vi "AMSClient.vi"() -> ()   [LabVIEW 2013]
uses:
  Controls/DB - Logon Info.ctl
  Controls/DB - Logon Extra Info.ctl
  Controls/Combo Box.ctl
  Controls/Enum - CMS State.ctl
  <vilib>/Utility/miscctls.llb/LVPointTypeDef.ctl
  <vilib>/Utility/miscctls.llb/LVRowAndColumnUnsignedTypeDef.ctl
  <vilib>/Utility/miscctls.llb/LVRowAndColumnTypeDef.ctl
  Controls/DB - [AMS].[Execute].[Message] ColNames.ctl
  <vilib>/Utility/miscctls.llb/LVDateTimeRec.ctl
  Controls/DB - [AMS].[Execute].[Message] Enum.ctl
  <vilib>/Utility/NIReport.llb/NI_report.lvclass
  Controls/DB - OpenClose.ctl
  Controls/DB - [AMS].[Execute].[EventLog] Enum.ctl
  Controls/DB - AMS Execute EventLog.ctl
  Controls/Global AMS.vi
  <vilib>/Utility/NIReport.llb/Append Text Table to Report (wrap).vi
  Controls/Global CMS.vi
  <vilib>/Utility/config.llb/Write Key (String).vi
  Controls/Message Code - Enum.ctl
  Controls/Enum - SRTRS State.ctl
  <vilib>/Utility/config.llb/NI_LVConfig.lvlib
panel:
  in  "Tab Footer":enum32{"Page 1"}(tab) caption="Tab Header"
  out "Current Time":string
  in  "Tab Header":enum32{"Page 1"}(tab)
  out "LogoName":picture
  in  "Close":bool
  out "Plant and Furnace Name":string="OneSubsea, Johor / BH0277."
  out "ApplicationName":string caption="[LogoName]"
  in  "Tab Body":T1(tab)=enum."Logon"
  out "Last Alive On":string
  out "Overall Status":bool caption="Engine Status"
  in  "Search":bool caption="Setup Save"
  in  "Max Record to Display":i32 caption="Max. Records To Display"
  in  "Ref Message No":string caption="Ref. Message No."
  in  "Message No":string caption="Message No."
  in  "Plant":T2
  in  "Email":T2
  in  "SMS":T2
  in  "Application ComboBox":T2 caption="Application"
  in  "To Date":timestamp caption="To" format="%<%Y-%m-%d>T"
  in  "From Date":timestamp caption="From" format="%<%Y-%m-%d>T"
  in  "Criteria [CaptionOnly]":string caption="Criteria"
  in  "Resend":bool caption="Setup Save"
  in  "Reprocess [CaptionOnly]":string caption="Reprocess"
  in  "Excel":bool caption="Setup Save"
  in  "Export To [CaptionOnly]":string caption="Export To"
  in  "List [CaptionOnly]":string caption="List"
  in  "Multicolumn Listbox":i32[](listbox)
  in  "MyTab":T3(tab)
  out "Toggle Search":bool=TRUE
  out "Property":errorcluster
  in  "CellBG Unused Cells":u32(colorbox)=16777238
  in  "CellBG ColHdrs":u32(colorbox)=11776947
  in  "Ascending":bool
  out "<CONDITIONS>":string="[MessageNo] >0"
  out "EnginePollIntInSec":i32
  in  "Time Target (s)":dbl=1.0
  out "Engine Alive":timestamp format="%<%I:%M:%S%3u %p\n%x>T"
  out "Engine Start":timestamp format="%<%I:%M:%S%3u %p\n%x>T"
  out "Engine Stop":timestamp format="%<%I:%M:%S%3u %p\n%x>T"
  out "Report":errorcluster
  out "Toggle Refresh MCListBox Colors":bool=TRUE
  out "Metrics:Code Size":u32=1762288 format="%#.3p"
  out "SubPanel Error":errorcluster
  out "Logon OK":bool
  in  "[TabUserAccess]":bool[](array[boolean])=[FALSE, FALSE, FALSE, FALSE, FALSE, FALSE, FALSE, FALSE, FALSE, FALSE, FALSE, FALSE, FALSE, FALSE, FALSE, FALSE, FALSE, FALSE, FALSE, FALSE]
  in  "Logon Extra":T4
  in  "Logon":T5
  out "Current VI's path":path
  out "Front Panel Window:State":T6(ring)
  out "Execution:State":T7(ring)
  out "Admin User UI":refnum<vi>
  out "Logon UI":refnum<vi>
  out "Config UI":refnum<vi>
  in  "Application":string="AMS"
  out "Max Rec to Display (Startup)":i32
  out "ini File":errorcluster
  out "LogonName Error":errorcluster
  out "Station":string
  out "Plant":string
  out "LabVIEW Directory Path":path
  out "Application:Name":string="LabVIEW.exe"
  out "[TimeZone] (Plant)":string
  out "[CmsServerTz] (CMS)":string
  out "TimeZone Diff (NA)":i32
  out "Plant and Furnace Name (B4 Logon)":string="OneSubsea, Johor / BH0277." caption="Plant and Furnace Name"
  out "Application Directory":path=path "C:/Users/CK/workspace/LabVIEW/Stress Relief Temperature Recording"
  out "Error Out":errorcluster
  out "Show Debug TAB":bool=TRUE caption="Show Debug Tab"
  out "Quit Flag":bool
  out "Close Flag":bool=TRUE
  out "Summary":errorcluster
  out "MHandler":errorcluster
  in  "DB - Logon":bool=TRUE
  out "File Version":string
  in  "Debug Close":bool caption="Close"
  # "User Details"
  # "System Status"
  # "Logon"
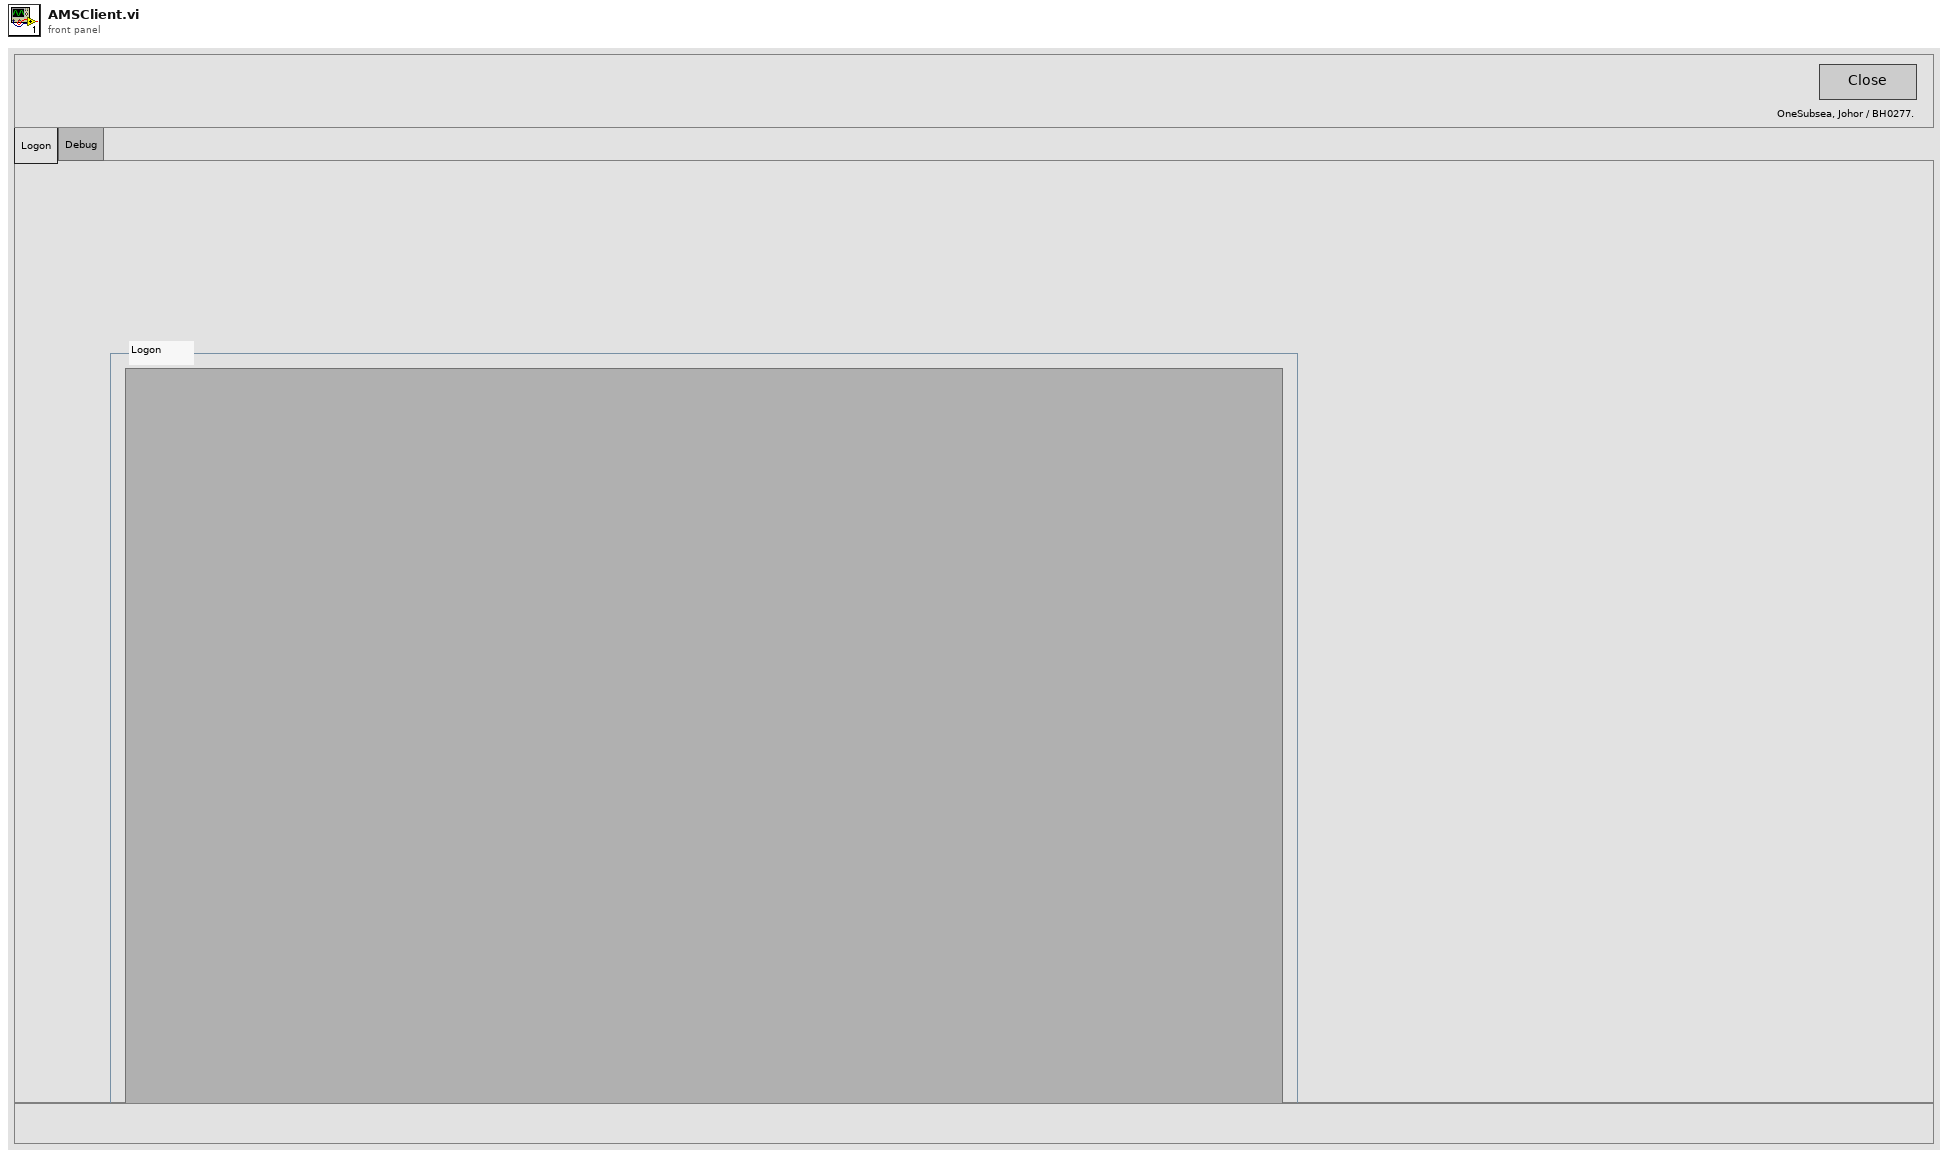
[diagram p1: front panel]
types:
  T1 = enum32{"Monitor", "Admin", "Config", "Logon", "Debug"}
  T2 = typedef "Combo Box.ctl" = string
  T3 = enum32{"Monitor", "SubPanel", "Settings", "Others", "DB"}
  T4 = typedef "DB - Logon Extra Info.ctl" = cluster{"Plant Name":string, "UserName":string, "Hostname [ClientName]":string, "IsUnicode":bool}
  T5 = typedef "DB - Logon Info.ctl" = cluster{"PlantID":string, "SystemID":string, "UserID":string, "DomainID":string, "LanguageID":string, "StationID":string}
  T6 = enum32{"Invalid", "Standard", "Closed", "Hidden", "Minimized", "Maximized"}
  T7 = enum32{"Bad", "Idle", "Run top level", "Running"}
  T8 = typedef "Enum - CMS State.ctl" = enum16{"READY TO START", "RUNNING Process", "QUIT"}
  T9 = enum16{"Always On", "Always Off", "Off While Running"}
  T10 = typedef "LVRowAndColumnUnsignedTypeDef.ctl" = cluster{"Row":u32, "Column":u32}
  T11 = typedef "LVPointTypeDef.ctl" = cluster{"Horizontal":i16, "Vertical":i16}
  T12 = typedef "DB - [AMS].[Execute].[Message] ColNames.ctl" = enum16{"[MessageNo]", "[LanguageId]", "[SoftwareSolutionId]", "[SoftwareSolutionName]", "[PlantId]", "[SystemId]", "[StationId]", "[MessageLogNo]", "[ReceivedOn]", "[MessageCode]", "[ShortDescription]", "[Message]", "[SmsMessage]", "[SuppMessage1]", "[SuppMessage2]", "[SuppMessage3]", "[TransactionNo]", "[TransactionRunNo]", "[MessageInitiator]", "[Remarks]", "[MsgCreatedOn]", "[IsToSendSms]", "[IsToSendEmail]", "[IsToSendCommMedium1]", "[IsToSendCommMedium2]", "[SmsContent]", "[EmailContent]", "[CommMed1Content]", "[CommMed2Content]", "[MobileNos]", "[EmailAddresses]", "[CommMedium1Ids]", "[CommMedium2Ids]", "[LastAttemptedCommMed]", "[LastAttemptedNo]", "[LastAttemptedOn]", "[IsSmsSent]", "[IsEmailSent]", "[IsCommMedium1Sent]", "[IsCommMedium2Sent]", "[OverallSentStatus]", "[StatusUpdatedOn]", "[IsArchived]"}
  T13 = typedef "LVRowAndColumnTypeDef.ctl" = cluster{"Row":i32, "Column":i32}
  T14 = cluster{"LogoFile":string, "Software Solution Name":string}
  T15 = typedef "Connection Information Cluster.ctl" = cluster{"Connection ":string, "Username":string, "Password":string}
  T16 = cluster{"Show LabVIEW Error":bool, "Show Debug Tab":bool, "Show Scrollbars":bool}
  T17 = typedef "imagedata.ctl" = cluster{"image type":i32, "image depth":i32, "image":u8[], "mask":u8[], "colors":u32[], "Rectangle":cluster{"left":i16, "top":i16, "right":i16, "bottom":i16}}
  T18 = typedef "Enum - SRTRS State.ctl" = enum16{"READY TO START", "START Recipe", "START Recovery", "BEGIN Process", "RUNNING Process", "END Process", "Spare Enum", "END Recipe", "ERROR Handling", "QUIT"}
  T19 = typedef "Message Code - Enum.ctl" = enum16{"<APP><I 100>", "<APP><E 101>", "<APP><I 110>", "<APP><W 111>", "<APP><I 112>", "<APP><W 113>", "<APP><I 114>", "<APP><I 115>", "<APP><I 116>", "<APP><W 117>", "<APP><I 120>", "<APP><W 121>", "<APP><E 122>", "<APP><W 130>", "<APP><W 131>", "<APP><W 132>", "<APP><W 133>", "<APP><W 134>", "<DB><I 150>", "<DB><I 151>", "<DB><W 152>", "<APP><I 200>", "<APP><I 201>", "<APP><W 202>", "<APP><E 203>", "<DB><I 300>", "<DB><I 301>", "<DB><W 302>", "<DB><I 305>", "<DB><I 306>", "<DB><W 307>", "<DB><W 310>", "<cRIO><I 400>", "<cRIO><W 401>", "<cRIO><I 402>", "<cRIO><W 403>", "<ET><I 500>", "<ET><W 501>", "<ET><I 600>", "<ET><W 601>", "<ET><E 602>", "<ET><I 610>", "<ET><W 611>", "<ET><E 612>"}
  T20 = typedef "DB - [AMS].[Execute].[Message] Enum.ctl" = enum16{"SELECT", "SELECT (Multi-Conditions)", "UPDATE", "RE-INSERT"}
  T21 = enum16{"maximized", "minimized", "normal", "no change"}
  T22 = enum16{"Standard Report", "HTML", "Word", "Excel"}
  T23 = typedef "LVDateTimeRec.ctl" = cluster{"fractional second":dbl, "second":i32, "minute":i32, "hour":i32, "day of month":i32, "month":i32, "year":i32, "day of week":i32, "day of year":i32, "DST":i32}
  T24 = typedef "DB - AMS Execute EventLog.ctl" = cluster{"EventType":string, "Source":string, "UserId":string, "Computer":string, "CreatedOn":string, "Remarks1":string}
  T25 = typedef "DB - OpenClose.ctl" = cluster{"Open":bool, "Close":bool}
  T26 = typedef "NI_LVConfig.lvlib/Config Data RefNum.ctl" = refnum<k1>
  T27 = typedef "DB - [AMS].[Execute].[EventLog] Enum.ctl" = enum16{"SELECT 'CreatedOn'", "SELECT 'LastMessageNo'", "INSERT"}
  T28 = typedef "NI_Database_API.lvlib/Conn ObjectReference.ctl" = refnum<k1>
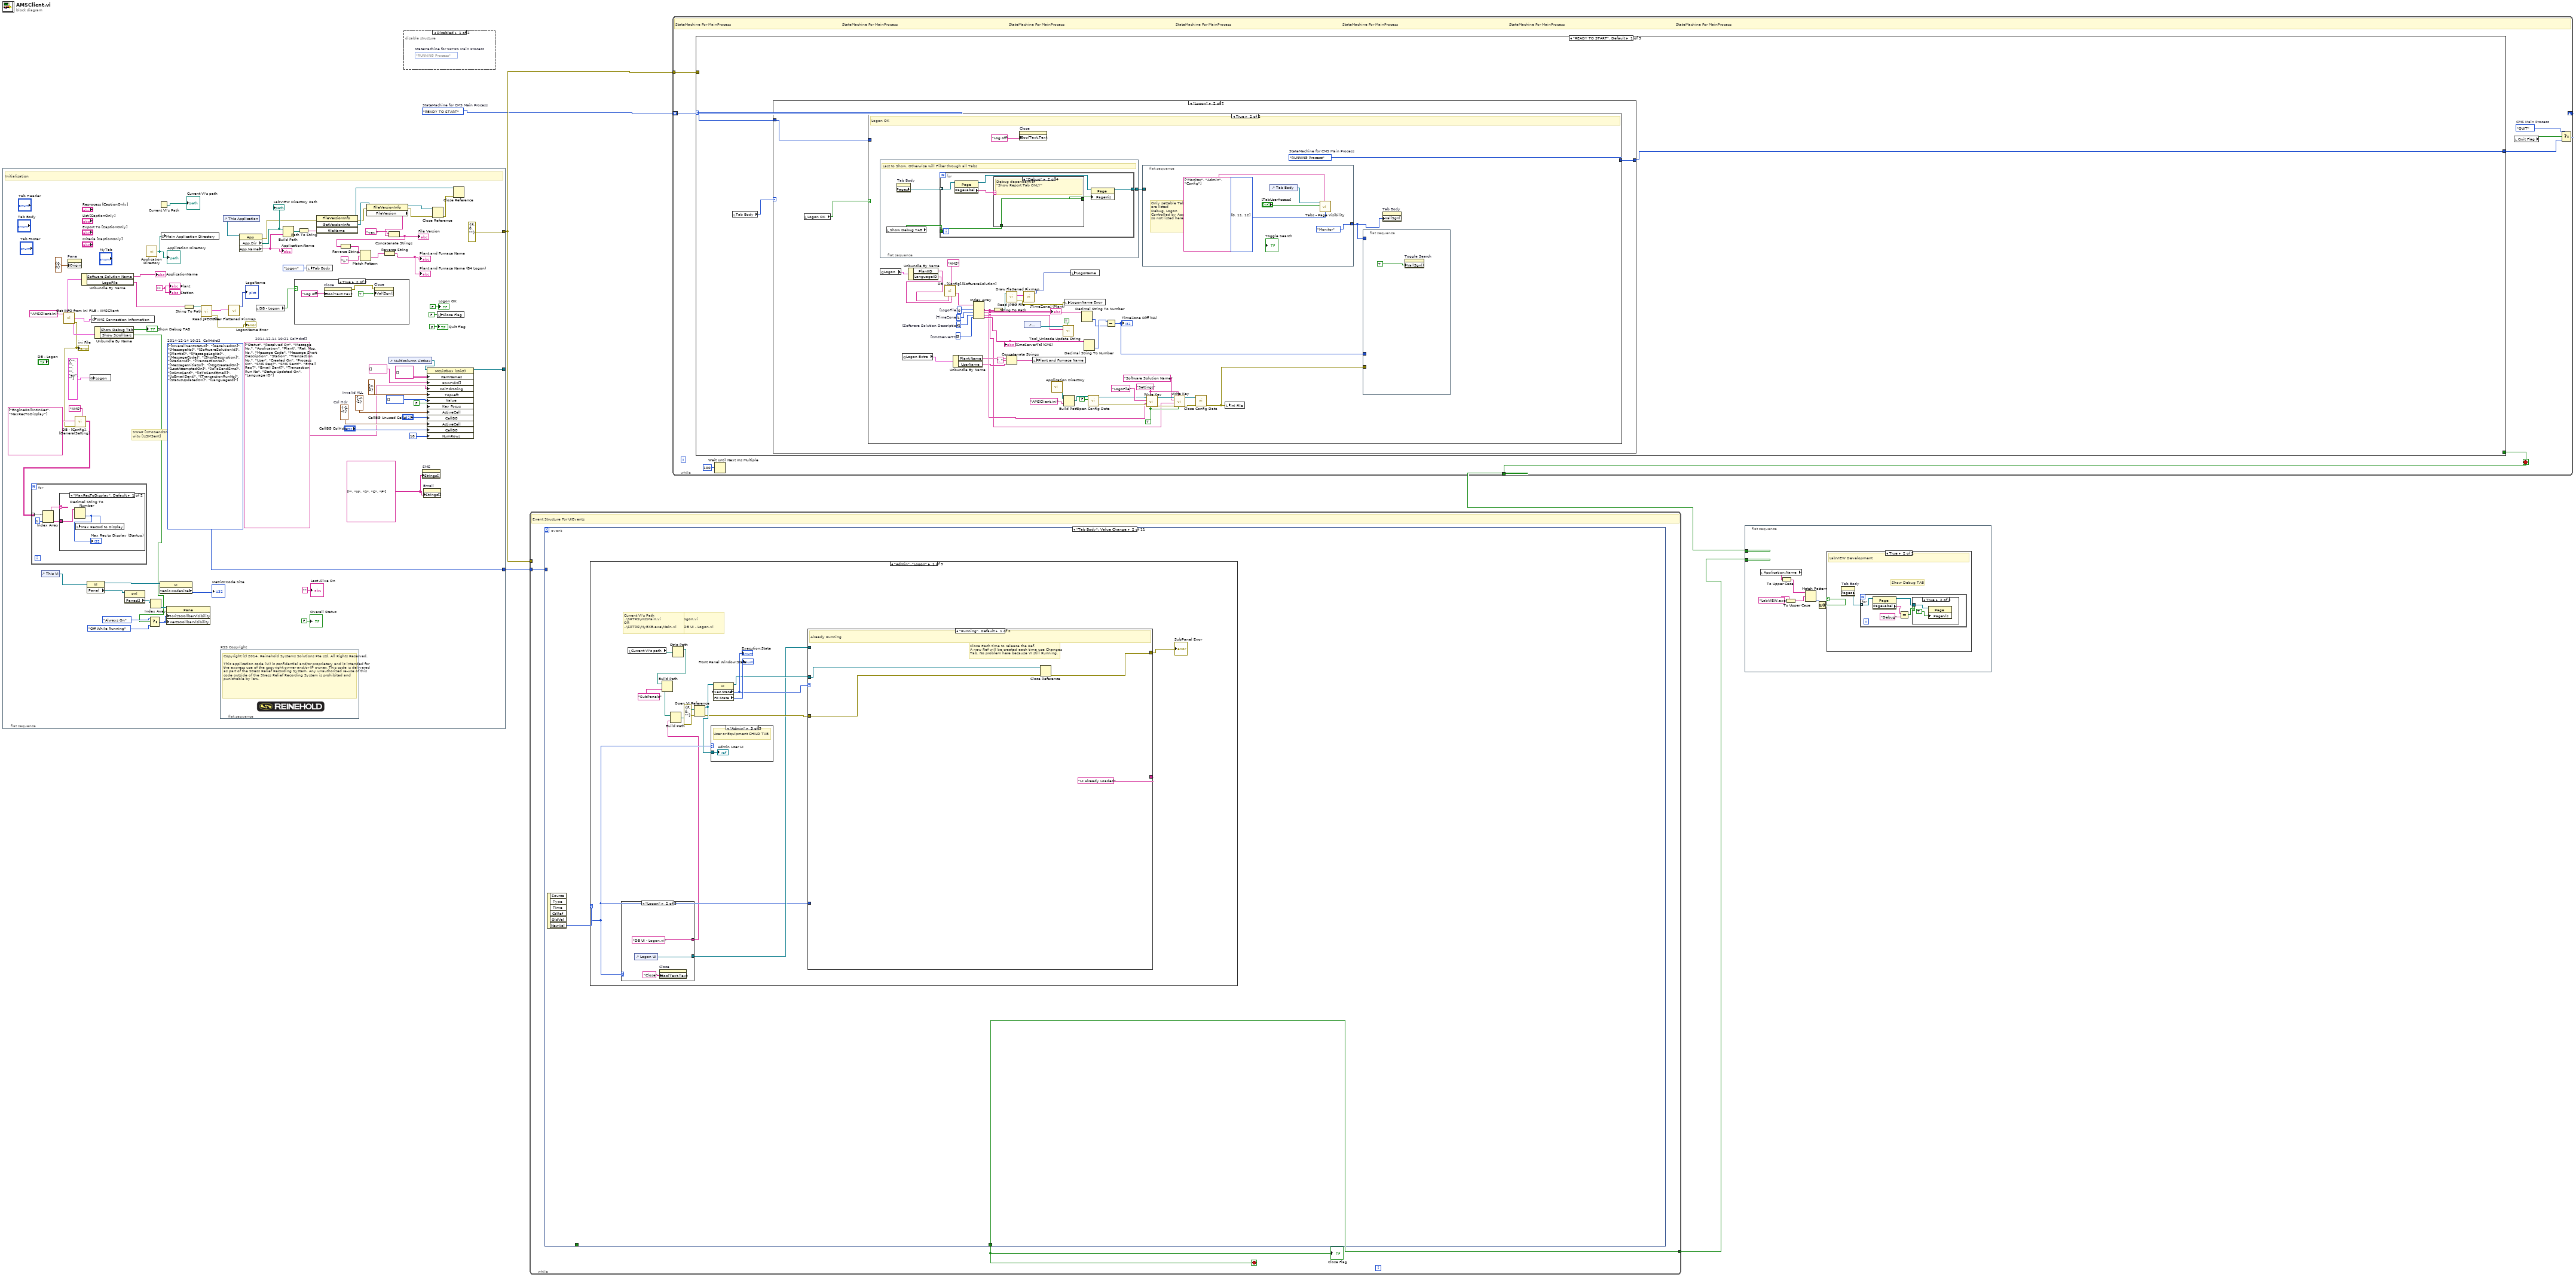
[diagram p0: block diagram]
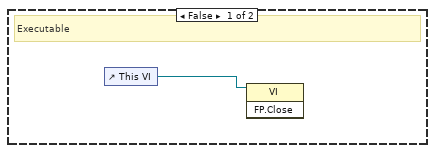
[diagram p2: hidden frame]
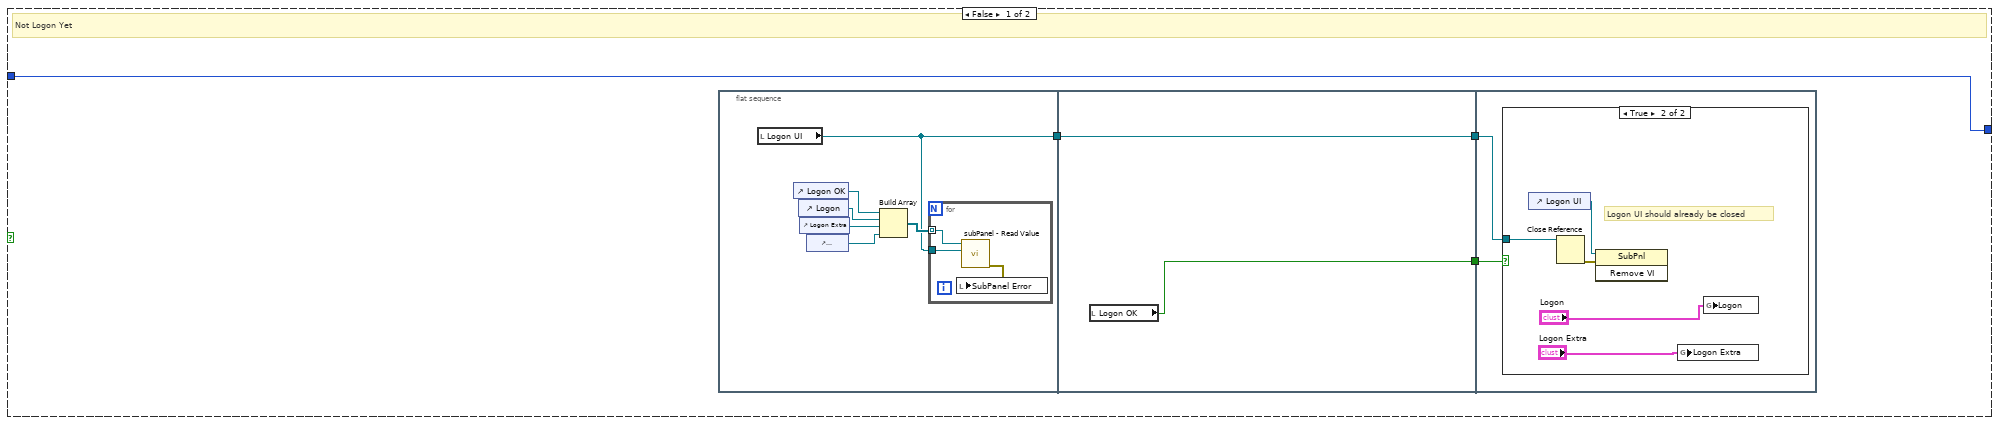
[diagram p6: hidden frame]
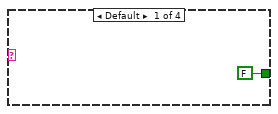
[diagram p8: hidden frame]
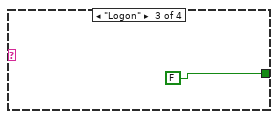
[diagram p9: hidden frame]
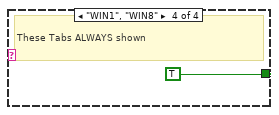
[diagram p10: hidden frame]
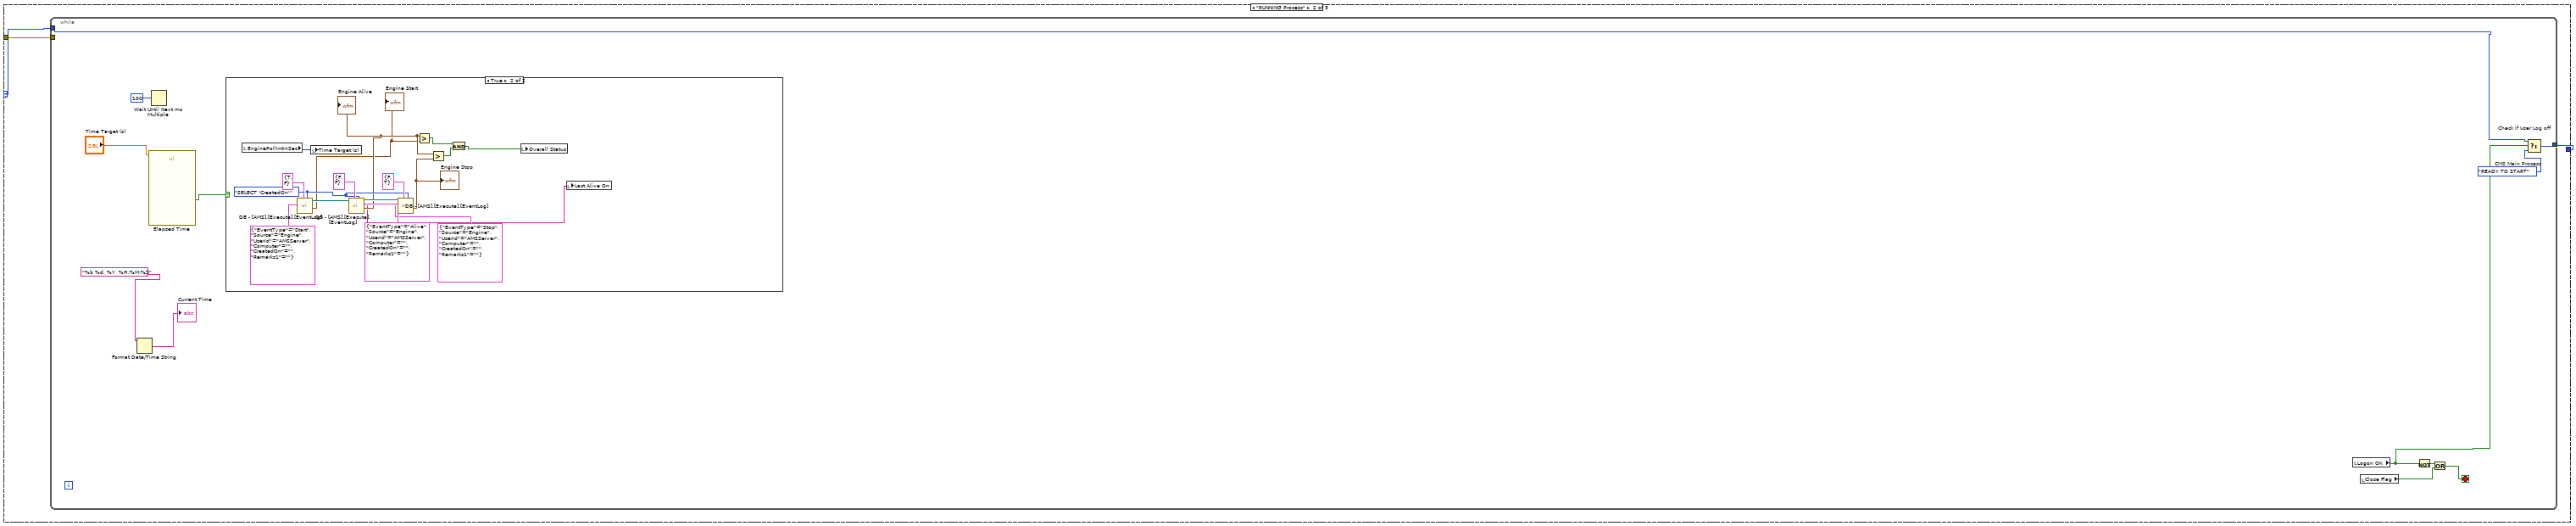
[diagram p11: hidden frame]
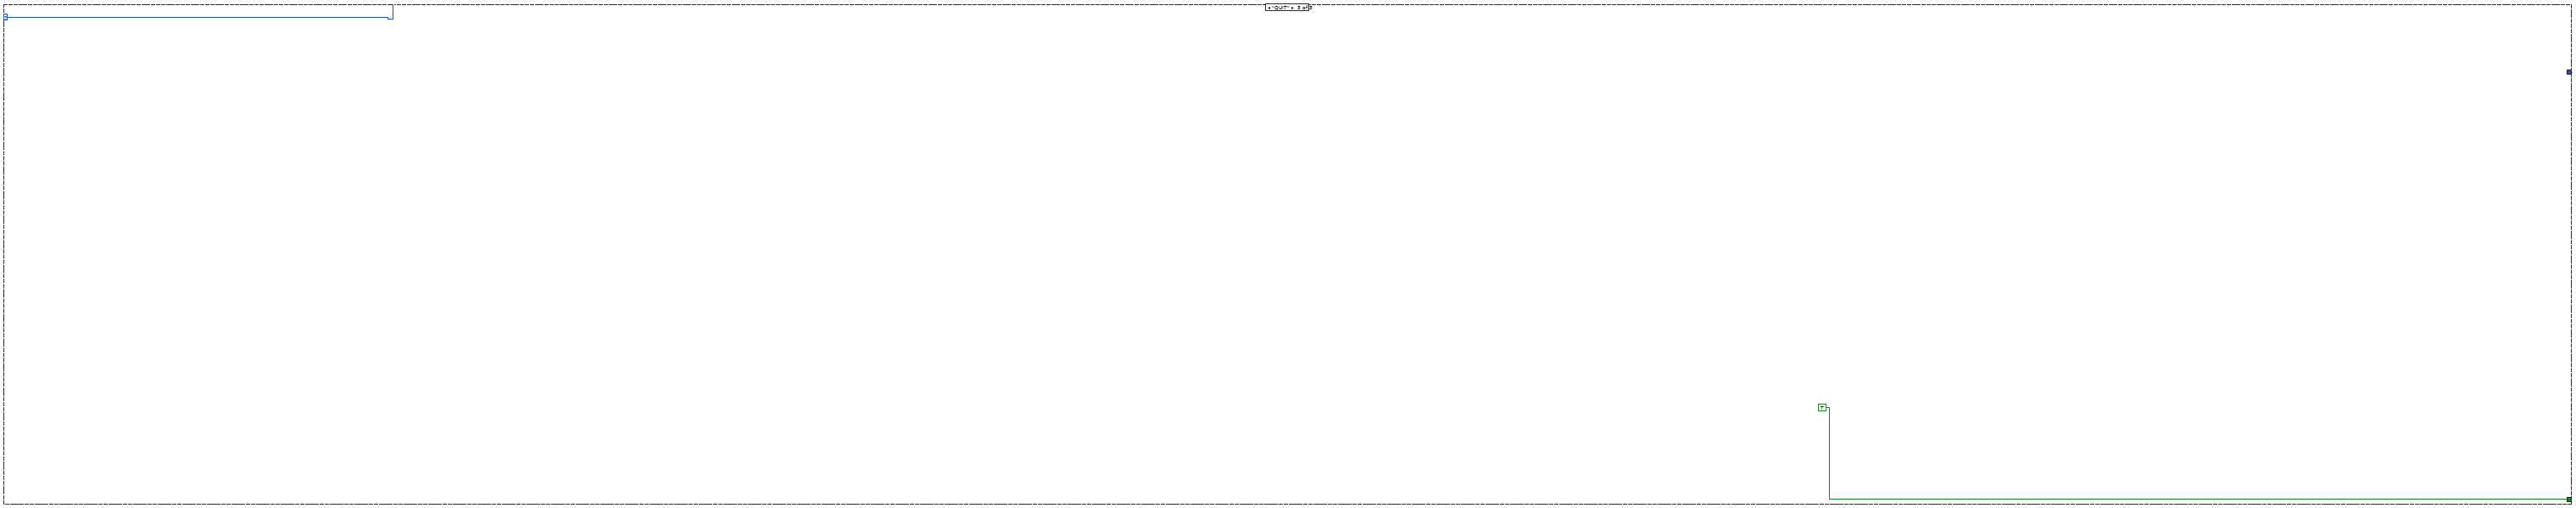
[diagram p13: hidden frame]
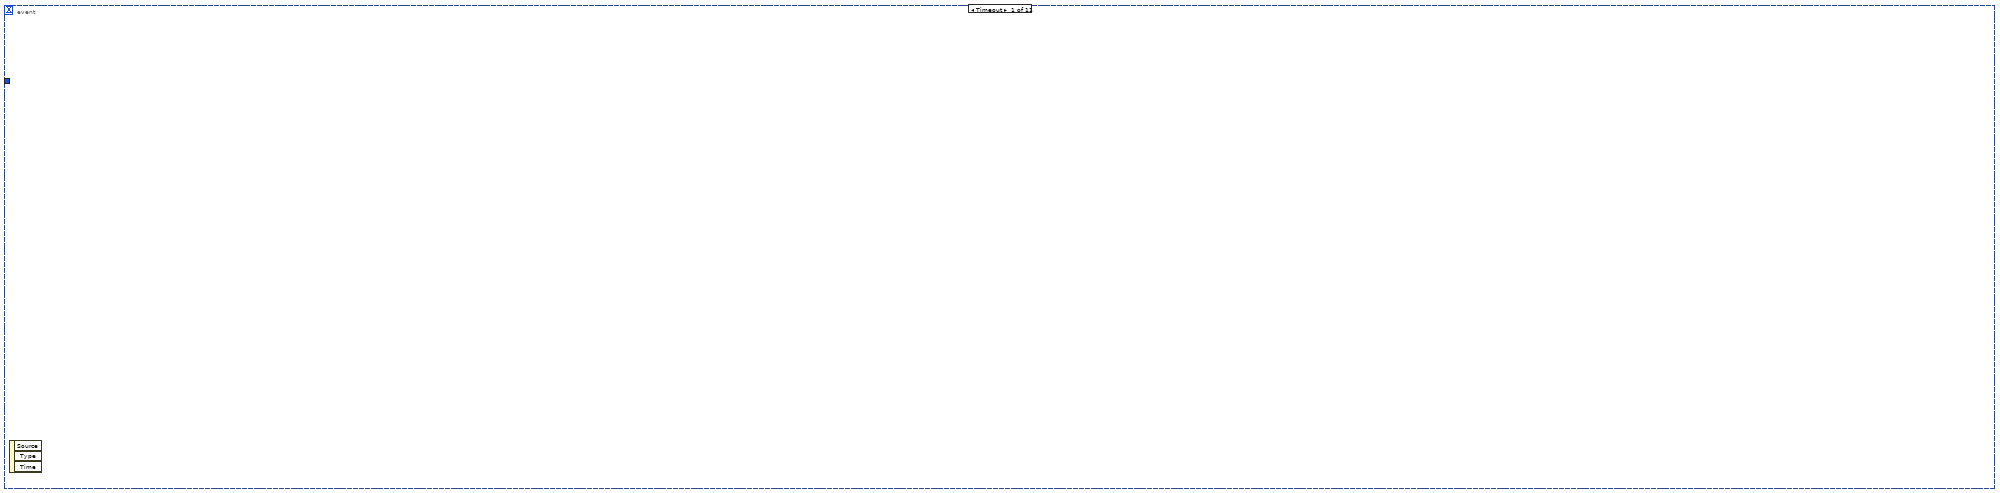
[diagram p14: hidden frame]
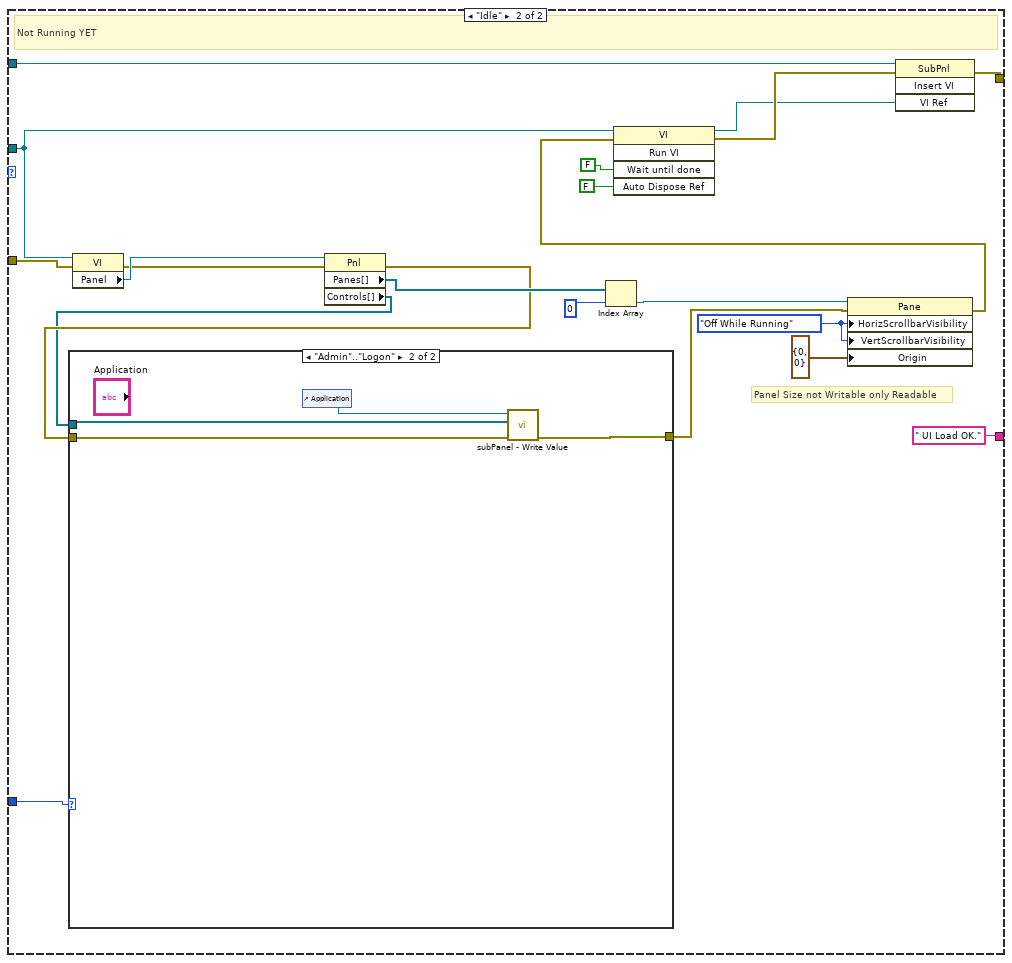
[diagram p15: hidden frame]
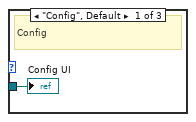
[diagram p17: hidden frame]
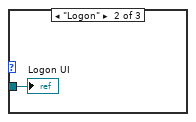
[diagram p18: hidden frame]
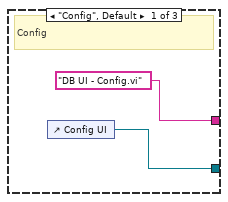
[diagram p19: hidden frame]
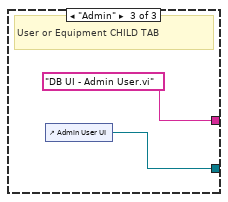
[diagram p20: hidden frame]
diagram:
  w4 = Enum_-_CMS_State."READY TO START"  # StateMachine for CMS Main Process
  n1 = flat-sequence {
    tunnel: [errorcluster {"status"=FALSE, "code"=0, "source"=""} ("error constant")] -> w5
    tunnel: [w36] -> _
    tunnel: [w33] -> w1
    frame #0 {
      w8 = ""
      w32 = string[] ["", "N", "R", "S", "F"]
      w33 = T12[] [enum."[OverallSentStatus]", enum."[ReceivedOn]", enum."[MessageNo]", enum."[SoftwareSolutionId]", enum."[PlantId]", enum."[MessageLogNo]", enum."[MessageCode]", enum."[ShortDescription]", enum."[StationId]", enum."[TransactionNo]", enum."[MessageInitiator]", enum."[MsgCreatedOn]", enum."[LastAttemptedOn]", enum."[IsToSendSms]", enum."[IsSmsSent]", enum."[IsToSendEmail]", enum."[IsEmailSent]", enum."[TransactionRunNo]", enum."[StatusUpdatedOn]", enum."[LanguageId]"] items=["[MessageNo]", "[LanguageId]", "[SoftwareSolutionId]", "[SoftwareSolutionName]", "[PlantId]", "[SystemId]", "[StationId]", "[MessageLogNo]", "[ReceivedOn]", "[MessageCode]", "[ShortDescription]", "[Message]", "[SmsMessage]", "[SuppMessage1]", "[SuppMessage2]", "[SuppMessage3]", "[TransactionNo]", "[TransactionRunNo]", "[MessageInitiator]", "[Remarks]", "[MsgCreatedOn]", "[IsToSendSms]", "[IsToSendEmail]", "[IsToSendCommMedium1]", "[IsToSendCommMedium2]", "[SmsContent]", "[EmailContent]", "[CommMed1Content]", "[CommMed2Content]", "[MobileNos]", "[EmailAddresses]", "[CommMedium1Ids]", "[CommMedium2Ids]", "[LastAttemptedCommMed]", "[LastAttemptedNo]", "[LastAttemptedOn]", "[IsSmsSent]", "[IsEmailSent]", "[IsCommMedium1Sent]", "[IsCommMedium2Sent]", "[OverallSentStatus]", "[StatusUpdatedOn]", "[IsArchived]"]  # 2014-12-14 10:21  ColHdrs[]
      w39 = T13 {"Row"=-1, "Column"=-2}  # Col Hdr
      w40 = T13 {"Row"=-2, "Column"=-2}  # Invalid ALL
      w31 = string[] ["Status", "Received On", "Message No.", "Application", "Plant", "Ref. Msg. No.", "Message Code", "Message Short Description", "Station", "Transaction No.", "User", "Created On", "Process On", "SMS Req?", "SMS Sent?", "Email Req?", "Email Sent?", "Transaction Run No", "Status Updated On", "Language ID"]  # 2014-12-14 10:21 ColHdrs[]
      # "SWAP [IsToSendSMS]\nwitu [IsSMSent]"
      # "Initialisation"
      n2 = control-ref of="This VI"() -> (w16:refnum<vi>)
      n3 = call "Get INFO from ini FILE - AMSClient.vi"("ini Name"="AMSClient.ini") -> ("Settings"=w69:T14, "AMS Connection Information"=w46:T15, "Settings Boolean"=w70:T16, "Error Out"=w6:errorcluster)  [unwired: 8 in, 3 out]
      "ini File" <- w6
      n4 = property on="Pane" class="Pane"("Origin"=T11 {"Horizontal"=0, "Vertical"=0}) -> ()  [unwired: 2 in, 2 out]
      n5 = call "DB - [Config].[GeneralSetting].vi"("Application"="AMS", "error in (no error)"=w6, "[SettingId] Values"=string[] ["EnginePollIntInSec", "MaxRecToDisplay"]) -> ("2D data"=w7:string[][])  [unwired: 6 in, 2 out]
      n6 = for {
        tunnel: w7 -> [w81] mode=indexing
        n7 = Index Array(array=w81, index #2=1 ("index")) -> (element #1=w80:string, element #2=w78:string)  [unwired: 1 in]
        n8 = case shown="\"MaxRecToDisplay\", Default" w80 {
          tunnel: w78 -> [w83 w85]
          frame "MaxRecToDisplay", Default {
            n9 = Decimal String To Number(string=w83) -> (number=w82:i32)  [unwired: 2 in, 1 out]
            "Max Rec to Display (Startup)" <- w82
            n10 = local write "Max Record to Display"(w82) -> ()
          }
          frame "EnginePollIntInSec" {
            n11 = Decimal String To Number(string=w85) -> (number=→"EnginePollIntInSec":i32)  [unwired: 2 in, 1 out]
          }
        }
      }
      n12 = Unbundle By Name(w69) -> ("Software Solution Name"=→"ApplicationName":string, "LogoFile"=w11:string)
      n13 = property class="VI"(reference=w16) -> (reference out=w22:refnum<vi>, "Panel"=w23:refnum<vi>)  [unwired: 1 in, 1 out]
      n14 = global write "Global AMS.vi" "Logon"(T5 {"PlantID"="", "SystemID"="", "UserID"="", "DomainID"="", "LanguageID"="en", "StationID"=""} ("Logon")) -> ()
      n15 = global write "Global AMS.vi" "AMS Connection Information"(w46) -> ()
      n16 = Unbundle By Name(w70) -> ("Show Debug Tab"=→"Show Debug TAB":bool, "Show Scrollbars"=w15:bool)
      n17 = property class="Pnl"(reference=w23) -> ("Panes[]"=w21:refnum<vi>[])  [unwired: 1 in, 2 out]
      n18 = call <vilib>:"Application Directory.vi"() -> ("Application Directory"=w14:path)
      "Application Directory" <- w14
      n19 = Select(t=T9."Always On" ("Vertical Scrollbar Visibility"), s=w15, f=T9."Off While Running" ("Vertical Scrollbar Visibility")) -> (s? t:f=w17:T9)
      n20 = Index Array(array=w21) -> (element=w20:refnum<vi>)  [unwired: 1 in]
      n21 = Current VI's Path() -> (path=→"Current VI's path":path)
      n22 = property class="VI"(reference=w22) -> ("Metric.CodeSize"=→"Metrics:Code Size":u32)  [unwired: 1 in, 2 out]
      n23 = global write "Global AMS.vi" "Main Application Directory"(w14) -> ()
      n24 = property class="Pane"(reference=w20, "HorizScrollbarVisibility"=w17, "VertScrollbarVisibility"=w17) -> ()  [unwired: 1 in, 2 out]
      n25 = String To Path(string=w11) -> (path=w13:path)
      n26 = call <vilib>:"Read JPEG File.vi"("path to JPEG file"=w13) -> ("error out"=→"LogonName Error":errorcluster, "image data"=w12:T17)  [unwired: 8 in, 1 out]
      n27 = flat-sequence "RSS Copyright" {
        frame #0 {
          # "Copyright (c) 2014, Reinehold Systems Solutions Pte Ltd. All Rights Reserved.\n\nThis application code (VI) is confidential and/or proprietary and is intended for the express use of the copyright owner and/or IP owner. This code is delivered as part of the Stress Relief Recording System. Any unauthorized re-use of this code outside of the Stress Relief Recording System is prohibited and punishable by law."
        }
      }
      n28 = control-ref of="This Application"() -> (w66:refnum<vi>)
      n29 = call <vilib>:"Draw Flattened Pixmap.vi"("image data"=w12) -> ("new picture"=→"LogoName":picture)  [unwired: 8 in]
      n30 = property class="App"(reference=w66) -> (error out=w59:errorcluster, "App.Dir"=w65:path, "App.Name"=w53:string)  [unwired: 1 in, 1 out]
      "LabVIEW Directory Path" <- w65
      "Application:Name" <- w53
      n31 = local read "DB - Logon"() -> (w73:bool)
      n32 = Build Path(base path=w65, name or relative path=w53) -> (appended path=w64:path)
      n33 = case shown="True" w73 {
        frame False {
        }
        frame True {
          n34 = property on="Close" class="Bool (strict)"("BoolText.Text"="Log off" ("Label.Text")) -> (error out=w86:errorcluster)  [unwired: 2 in, 1 out]
          n35 = property on="Close" class="Bool (strict)"(error in=w86, "Val(Sgnl)"=TRUE ("Value (Signaling)")) -> ()  [unwired: 1 in, 2 out]
        }
      }
      n36 = Path To String(path=w64) -> (string=w63:string)
      n37 = local write "Tab Body"(T1."Logon" ("Tab Body")) -> ()
      n38 = invoke class="FileVersionInfo" method="GetVersionInfo"(error in=w59, "fileName"=w63) -> (reference out=w60:refnum<k24>, error out=w58:errorcluster, "GetVersionInfo"=w62:refnum<k24>)  [unwired: 2 in, 1 out]
      n39 = property class="FileVersionInfo"(reference=w62, error in=w58) -> (reference out=w61:refnum<k24>, error out=w57:errorcluster, "FileVersion"=w54:string)
      n40 = Concatenate Strings("ver. ", w54) -> (w49:string)
      "File Version" <- w49
      n41 = Reverse String(1:w49) -> (0:w50:string)
      n42 = Match Pattern(string=w50, regular expression="\\." ("search string")) -> (after substring=w52:string)  [unwired: 1 in, 3 out]
      n43 = Reverse String(1:w52) -> (0:→"Plant and Furnace Name" →"Plant and Furnace Name (B4 Logon)":string)
      n44 = control-ref of="Multicolumn Listbox"() -> (w35:refnum<vi>)
      n45 = property on="SMS" class="CmbBox (strict)"("Strings[]"=w32) -> ()  [unwired: 2 in, 2 out]
      n46 = property on="Email" class="CmbBox (strict)"("Strings[]"=w32) -> ()  [unwired: 2 in, 2 out]
      n47 = property on="Property Node" class="MCListbox (strict)"(reference=w35, "ItemNames"=string[][] [] ("Item Names"), "RowHdrs[]"=string[] [] ("Item Names"), "ColHdrString"=w31, "TopLeft"=T10 {"Row"=0, "Column"=0} ("Top Left Visible Cell"), "Value"=i32[] [], "Key Focus"=FALSE, "ActiveCell"=w40, "CellBG"="CellBG Unused Cells", "ActiveCell"=w39, "CellBG"="CellBG ColHdrs", "NumRows"=u32 18 ("Number of Rows")) -> (reference out=w36:refnum<vi>)  [unwired: 1 in, 1 out]
      n48 = Close Reference(reference=w61, error in (no error)=w57) -> (error out=w56:errorcluster)
      n49 = local write "Close Flag"(FALSE ("Close Flag")) -> ()
      n50 = Close Reference(reference=w60, error in (no error)=w56) -> ()  [unwired: 1 out]
      "Logon OK" <- FALSE ("Logon OK")
      "Plant" <- w8
      "Station" <- w8
      "Quit Flag" <- FALSE ("Quit Flag")
      "Last Alive On" <- "" ("Last Alive On")
      "Overall Status" <- FALSE ("Overall Status")
    }
  }
  n51 = disable-structure shown="Disabled" {
    frame Disabled {
      (unwired) Enum_-_SRTRS_State."RUNNING Process"  # StateMachine for SRTRS Main Process
    }
    frame Enabled {
    }
  }
  n52 = while {
    tunnel: w5 -> [_]
    tunnel: [w90] -> w2
    tunnel: w1 -> [w89]
    stop <- w90 stop-if-true
    # "Event Structure For UIEvents"
    n53 = event shown="[1] \"Tab Body\": Value Change" {
      selector: _ -> [_ _ _ _ _ _ _ _ _ _ _]
      dyn-events: _ -> [_ _ _ _ _ _ _ _ _ _ _]
      timeout: _ -> [_ _ _ _ _ _ _ _ _ _ _]
      tunnel: [_ _ w169 _ _ _ _ _ _ _ _] -> _
      tunnel: [_ _ w167 _ _ _ _ _ _ _ _] -> w90
      tunnel: w89 -> [_ _ _ _ _ _ w280 _ w360 _ w450]
      event Timeout {
        n54 = event-data() -> ()  [unwired: 1 in, 3 out]
      }
      event "Tab Body": Value Change {
        n55 = event-data() -> ("NewVal"=w91:T1)  [unwired: 1 in, 5 out]
        n56 = case shown="\"Admin\"..\"Logon\"" w91 {
          selector: w91 -> [w95 _ _]
          frame "Admin".."Logon" {
            # "SubPanel VI's Path\n..\\SRTRS\\VIs\\SubPanels\\DB UI - Logon.vi\nOR \n..\\SRTRS\\MyEXE.exe\\SubPanels\\DB UI - Logon.vi"
            # "Current VI's Path\n..\\SRTRS\\VIs\\Main.vi\nOR \n..\\SRTRS\\MyEXE.exe\\Main.vi"
            n57 = case shown="\"Logon\"" w95 {
              tunnel: [w140 w142 w146] -> w96
              tunnel: ["DB UI - Config.vi" ("name or relative path") "DB UI - Logon.vi" ("name or relative path") "DB UI - Admin User.vi" ("name or relative path")] -> w94
              frame "Config", Default {
                # "Config"
                n58 = control-ref of="Config UI"() -> (w140:refnum<vi>)
              }
              frame "Logon" {
                n59 = control-ref of="Logon UI"() -> (w142:refnum<vi>)
                n60 = property on="Close" class="Bool (strict)"("BoolText.Text"="Close") -> ()  [unwired: 2 in, 2 out]
              }
              frame "Admin" {
                # "User or Equipment CHILD TAB"
                n61 = control-ref of="Admin User UI"() -> (w146:refnum<vi>)
              }
            }
            n62 = local read "Current VI's path"() -> (w103:path)
            n63 = Strip Path(path=w103) -> (stripped path=w106:path)  [unwired: 1 out]
            n64 = Build Path(base path=w106, name or relative path="SubPanels") -> (appended path=w104:path)
            n65 = Build Path(base path=w104, name or relative path=w94) -> (appended path=w100:path)
            n66 = Open VI Reference(vi path=w100, error in (no error)=errorcluster {"status"=FALSE, "code"=0, "source"=""}) -> (vi reference=w102:refnum<vi>, error out=w97:errorcluster)  [unwired: 4 in]
            n67 = case shown="\"Admin\"" w95 {
              tunnel: w102 -> [w137 w138 w139]
              frame "Config", Default {
                # "Config"
                "Config UI" <- w137
              }
              frame "Logon" {
                "Logon UI" <- w138
              }
              frame "Admin" {
                # "User or Equipment CHILD TAB"
                "Admin User UI" <- w139
              }
            }
            n68 = property class="VI"(reference=w102) -> (reference out=w98:refnum<vi>, "Exec.State"=w99:T7, "FP.State"=→"Front Panel Window:State":T6)  [unwired: 1 in, 1 out]
            "Execution:State" <- w99
            n69 = case shown="\"Running\", Default" w99 {
              tunnel: w97 -> [w108 w130]
              tunnel: [w107 w128] -> w92
              tunnel: w98 -> [w109 w123]
              tunnel: ["UI Already Loaded" ("string") " UI Load OK." ("string")] -> _
              tunnel: w96 -> [_ w121]
              tunnel: w95 -> [_ w115]
              frame "Running", Default {
                # "Close Each time to release the Ref.\nA new Ref will be created each time use Changes\nTab. No problem here because VI still Running."
                # "Already Running"
                n70 = Close Reference(reference=w109, error in (no error)=w108) -> (error out=w107:errorcluster)
              }
              frame "Idle" {
                w126 = T9."Off While Running" ("Horizontal Scrollbar Visibility")
                # "Panel Size not Writable only Readable"
                # "Not Running YET"
                n71 = property class="VI"(reference=w123, error in=w130) -> (error out=w129:errorcluster, "Panel"=w131:refnum<vi>)  [unwired: 1 out]
                n72 = property class="Pnl"(reference=w131, error in=w129) -> (error out=w114:errorcluster, "Panes[]"=w116:refnum<vi>[], "Controls[]"=w113:refnum<vi>[])  [unwired: 1 out]
                n73 = case shown="\"Admin\"..\"Logon\"" w115 {
                  tunnel: w113 -> [_ w133]
                  tunnel: [w132 w135] -> w112
                  tunnel: w114 -> [w132 w134]
                  frame "Monitor", Default {
                  }
                  frame "Admin".."Logon" {
                    n74 = control-ref of="Application"() -> (w136:refnum<vi>)
                    n75 = call "subPanel - Write Value.vi"("Error In"=w134, "CtlRef Controls[]"=w133, "Pnl Control"=w136) -> ("Error Out"=w135:errorcluster)  [unwired: 6 in, 2 out]
                  }
                }
                n76 = Index Array(array=w116, index=0) -> (element=w124:refnum<vi>)
                n77 = property class="Pane"(reference=w124, error in=w112, "HorizScrollbarVisibility"=w126, "VertScrollbarVisibility"=w126, "Origin"=T11 {"Horizontal"=0, "Vertical"=0}) -> (error out=w111:errorcluster)  [unwired: 1 out]
                n78 = invoke class="VI" method="Run VI"(reference=w123, error in=w111, "Wait until done"=FALSE ("Wait Until Done"), "Auto Dispose Ref"=FALSE ("Auto Dispose Reference")) -> (reference out=w117:refnum<vi>, error out=w118:errorcluster)  [unwired: 1 in, 3 out]
                n79 = invoke on="Invoke Node" class="SubPnl" method="Insert VI"(reference=w121, error in=w118, "VI Ref"=w117) -> (error out=w128:errorcluster)  [unwired: 1 in, 3 out]
              }
            }
            "SubPanel Error" <- w92
          }
          frame "Monitor" {
            w154 = T23 {"fractional second"=0.0, "second"=0, "minute"=0, "hour"=0, "day of month"=0, "month"=0, "year"=0, "day of week"=0, "day of year"=0, "DST"=0} ("date time rec")
            # "Set 1 day b4 and today"
            n80 = Get Date/Time In Seconds() -> (seconds since 1Jan1904=w153:timestamp)
            n81 = Multiply(x=60, y=60) -> (x*y=w164:i32)
            n82 = Multiply(x=w164, y=24) -> (x*y=w162:i32)
            n83 = Subtract(x=w153, y=w162) -> (x-y=w161:timestamp)
            n84 = Seconds To Date/Time(time stamp (now)=w153) -> (date time rec=w152:T23)  [unwired: 1 in]
            n85 = Seconds To Date/Time(time stamp (now)=w161) -> (date time rec=w160:T23)  [unwired: 1 in]
            n86 = Unbundle By Name(w152) -> ("year"=w151:i32, "month"=w150:i32, "day of month"=w149:i32)
            n87 = Unbundle By Name(w160) -> ("year"=w158:i32, "month"=w157:i32, "day of month"=w156:i32)
            n88 = Bundle By Name(cluster=w154, "year"=w158, "month"=w157, "day of month"=w156) -> (w159:T23)
            n89 = Bundle By Name(cluster=w154, "year"=w151, "month"=w150, "day of month"=w149) -> (w148:T23)
            n90 = Date/Time To Seconds(2:w148) -> (0:w147:timestamp)  [unwired: 1 in]
            n91 = Date/Time To Seconds(2:w159) -> (0:w155:timestamp)  [unwired: 1 in]
            n92 = local write "To Date"(w147) -> ()
            n93 = local write "From Date"(w155) -> ()
          }
          frame Default {
          }
        }
      }
      event "Close", "Debug Close": Value Change {
        n94 = event-data() -> ("NewVal"=w169:bool)  [unwired: 1 in, 5 out]
        n95 = case shown="False" "Debug Close" {
          tunnel: [w171 w251] -> w167
          frame False {
            # "Close OR Log off"
            n96 = property on="Close" class="Bool (strict)"() -> ("BoolText.Text"=w170:string)  [unwired: 2 in, 2 out]
            n97 = case shown="\"Log off\", Default" w170 {
              tunnel: [FALSE ("T button?") w242] -> w171
              frame "Log off", Default {
                n98 = First Call?() -> (First Call?: T/F=w173:bool)
                n99 = case shown="False" w173 {
                  tunnel: [w178 TRUE ("T button?")] -> w174
                  frame False {
                    # "Prompt on subsequent Log off"
                    n100 = call "Msgbox - Message Handler.vi"("Application (Default SRTRS)"="AMS", "Short Description (When DB Not Available)"="Log off Application.", "Description (When DB Not Available)"="All unsaved data will be lost. Do you want to proceed Logoff?", "<.?....> Message Code"="<W 001>") -> ("MHandler Error"=→"MHandler":errorcluster, "OK Out"=w178:bool)  [unwired: 5 in, 1 out]
                  }
                  frame True {
                    (unwired) "1st Startup." ("string")
                    # "1st Startup, no prompt"
                  }
                }
                n101 = local write "Close"(FALSE ("Quit")) -> ()
                n102 = case shown="True" w174 {
                  frame False {
                  }
                  frame True {
                    # "Need to Stop\nthe {Running Process}\nLoop"
                    # "Log off CONFIRMED"
                    n103 = flat-sequence {
                      tunnel: [errorcluster {"status"=FALSE, "code"=0, "source"=""} ("error constant")] -> w188
                      frame #0 {
                        w220 = ""
                        w227 = T13 {"Row"=-1, "Column"=-2}  # Col Hdr
                        w228 = T13 {"Row"=-2, "Column"=-2}  # Invalid ALL
                        w239 = ""
                        n104 = local read "CellBG ColHdrs"() -> (w222:u32)
                        n105 = local read "Plant and Furnace Name (B4 Logon)"() -> (w236:string)
                        n106 = global read "Global AMS.vi" "Logon"() -> (w235:T5)
                        n107 = local read "Max Rec to Display (Startup)"() -> (w219:i32)
                        n108 = global read "Global AMS.vi" "Logon Extra"() -> (w233:T4)
                        n109 = Bundle By Name(cluster=w235, "UserID"=w239) -> (w234:T5)
                        n110 = Bundle By Name(cluster=w233, "UserName"=w239) -> (w232:T4)
                        n111 = local read "CellBG Unused Cells"() -> (w221:u32)
                        n112 = local write "Application ComboBox"(w220) -> ()
                        n113 = local write "SMS"(w220) -> ()
                        n114 = local write "Plant"(w220) -> ()
                        n115 = local write "Email"(w220) -> ()
                        n116 = control-ref of="Multicolumn Listbox"() -> (w226:refnum<vi>)
                        n117 = local write "Max Record to Display"(w219) -> ()
                        n118 = local write "Plant and Furnace Name"(w236) -> ()
                        n119 = local write "Ref Message No"(w220) -> ()
                        n120 = local write "Logon OK"(FALSE ("Logon OK")) -> ()
                        n121 = local write "Message No"(w220) -> ()
                        n122 = global write "Global AMS.vi" "Logon Extra"(w232) -> ()
                        n123 = property on="Property Node" class="MCListbox (strict)"(reference=w226, "ItemNames"=string[][] [] ("Item Names"), "RowHdrs[]"=string[] [] ("Item Names"), "TopLeft"=T10 {"Row"=0, "Column"=0} ("Top Left Visible Cell"), "Value"=i32[] [], "Key Focus"=FALSE, "ActiveCell"=w228, "CellBG"=w221, "ActiveCell"=w227, "CellBG"=w222, "NumRows"=u32 18 ("Number of Rows")) -> ()  [unwired: 1 in, 2 out]
                        n124 = global write "Global AMS.vi" "Logon"(w234) -> ()
                      }
                    }
                    n125 = local read "DB - Logon"() -> (w186:bool)
                    n126 = local read "Show Debug TAB"() -> (w187:bool)
                    n127 = property on="Tab Body" class="TabCtl (strict)"() -> ("Pages"=w189:refnum<vi>[])  [unwired: 2 in, 2 out]
                    n128 = case shown="True" w186 {
                      tunnel: w187 -> [w193 w207]
                      tunnel: w189 -> [w192 w206]
                      tunnel: w188 -> [w191 w204]
                      tunnel: [w190 w205] -> w185
                      frame False {
                        # "No DB"
                        n129 = for {
                          tunnel: w192 -> [w201] mode=indexing
                          tunnel: w193 -> [w200]
                          tunnel: w191 -> [w196]
                          tunnel: [w195] -> w190
                          (unwired) "Debug" ("y")
                          n130 = property class="Page"(reference=w201, error in=w196) -> (reference out=w197:refnum<vi>, error out=w194:errorcluster, "PageLabel"=w199:string)
                          n131 = case shown="\"Debug\"" w199 {
                            tunnel: w200 -> [w202 _]
                            tunnel: [w202 TRUE] -> w198
                            frame "Debug" {
                              # "Debug dependent of \n\"Show Debug Tab ONLY\""
                            }
                            frame Default {
                              # "These Tabs ALWAYS shown"
                            }
                          }
                          n132 = property class="Page"(reference=w197, error in=w194, "PageVis"=w198) -> (error out=w195:errorcluster)  [unwired: 1 out]
                        }
                      }
                      frame True {
                        # "Use DB to Logon"
                        n133 = for {
                          tunnel: w206 -> [w215] mode=indexing
                          tunnel: w207 -> [w214]
                          tunnel: [w210] -> w205
                          tunnel: w204 -> [w208]
                          (unwired) "Debug" ("y")
                          n134 = property class="Page"(reference=w215, error in=w208) -> (reference out=w211:refnum<vi>, error out=w209:errorcluster, "PageLabel"=w213:string)
                          n135 = case shown="\"Logon\"" w213 {
                            tunnel: w214 -> [_ w217 _]
                            tunnel: [FALSE ("Show Debug Tab") w217 TRUE] -> w212
                            frame Default {
                              # "All\nthese TAB will be hidden"
                            }
                            frame "Debug" {
                              # "Show Debug?"
                            }
                            frame "Logon" {
                              # "These Tabs ALWAYS shown"
                            }
                          }
                          n136 = property class="Page"(reference=w211, error in=w209, "PageVis"=w212) -> (error out=w210:errorcluster)  [unwired: 1 out]
                        }
                      }
                    }
                    n137 = property on="Tab Body" class="TabCtl (strict)"(error in=w185, "Val(Sgnl)"=T1."Logon" ("Value (Signaling)")) -> (error out=→"Error Out":errorcluster)  [unwired: 1 in, 1 out]
                  }
                }
              }
              frame "Close" {
                n138 = call "Msgbox - Message Handler.vi"("Application (Default SRTRS)"="CMS", "Short Description (When DB Not Available)"="Close Application", "Description (When DB Not Available)"="Confirm close Application?", "<.?....> Message Code"="<W 104>") -> ("MHandler Error"=w241:errorcluster, "OK Out"=w242:bool)  [unwired: 5 in, 1 out]
                n139 = local write "Quit Flag"(w242) -> ()
                n140 = local write "MHandler"(w241) -> ()
                n141 = flat-sequence {
                  tunnel: [w248] -> w247
                  tunnel: "Close" -> [w248]
                  tunnel: w247 -> [_]
                  frame #0 {
                    n142 = Wait (ms)(milliseconds to wait=u32 100) -> ()  [unwired: 1 out]
                  }
                  frame #1 {
                    n143 = local write "Close"(FALSE ("Quit")) -> ()
                  }
                }
              }
            }
          }
          frame True {
            # "Debug Close"
            n144 = flat-sequence {
              tunnel: [w252] -> w251
              frame #0 {
                w252 = TRUE ("T button?")
                n145 = local write "Quit Flag"(w252) -> ()
              }
              frame #1 {
                n146 = Wait Until Next ms Multiple(millisecond multiple=u32 200) -> ()  [unwired: 1 out]
              }
              frame #2 {
                n147 = disable-structure shown="Disabled" {
                  frame Disabled {
                    n148 = call "Msgbox - Format Message.vi"("Message"="{Debug CLOSE}" ("string"), "Message Code\n2014-10-01"=Message_Code_-_Enum."<APP><W 113>" ("Message Code\n2014-10-01")) -> ("Message"=w254:string)  [unwired: 8 in, 1 out]
                    n149 = call "Queue - EnQueue to MessageQ.vi"("Message"=w254) -> ()  [unwired: 10 in, 1 out]
                  }
                  frame Enabled {
                  }
                }
              }
            }
          }
        }
      }
      event "Tab Body": Shortcut Menu Activation? {
        # "Allow user to Re-Enable [ToggleTab] \nif it was already disabled"
        n150 = event-data() -> ()  [unwired: 1 in, 7 out]
        n151 = disable-structure shown="Disabled" {
          frame Disabled {
            w257 = "Toggle Between Tabs" ("item tag")
            n152 = Set Menu Item Info(7:w257, 10:w257) -> ()  [unwired: 5 in, 2 out]
          }
          frame Enabled {
          }
        }
        n153 = event-data() -> ()  [unwired: 2 in, 1 out]
      }
      event "Application": Mouse Down? {
        n154 = event-data() -> ()  [unwired: 1 in, 8 out]
        n155 = event-data() -> ()  [unwired: 2 in, 1 out]
      }
      event "Multicolumn Listbox": Mouse Up {
        n156 = event-data() -> ("CtlRef"=w261:refnum<vi>)  [unwired: 1 in, 7 out]
        n157 = property class="MCListbox (strict)"(reference=w261) -> (reference out=w260:refnum<vi>, "Value"=w259:i32[])  [unwired: 1 in, 1 out]
        n158 = Empty Array?(array=w259) -> (empty?=w258:bool)
        n159 = case shown="True" w258 {
          tunnel: w260 -> [_ w262]
          frame False {
            # "A row is Clicked"
          }
          frame True {
            # "Row not Clicked.. Must be Col Hdr"
            n160 = control-ref of="Ascending"() -> (w264:refnum<vi>)
            n161 = call "MCListbox Event - Sort Table (Array Selection).vi"("Clicked Color"=u32 16777216, "Sort Order Boolean Ref"=w264, "MCListBox Ref"=w262) -> ("ItemNames"=w263:string[][])  [unwired: 8 in]
            n162 = flat-sequence {
              tunnel: w263 -> [_]
              frame #0 {
                n163 = property on="Toggle Refresh MCListBox Colors" class="Bool (strict)"() -> (error out=w267:errorcluster, "Value"=w269:bool)  [unwired: 2 in, 1 out]
                n164 = Not(x=w269) -> (.not. x?=w268:bool)
                n165 = property on="Toggle Refresh MCListBox Colors" class="Bool (strict)"(error in=w267, "Val(Sgnl)"=w268) -> (error out=w266:errorcluster)  [unwired: 1 in, 1 out]
                n166 = local write "Property"(w266) -> ()
              }
            }
          }
        }
      }
      event "Toggle Search": Value Change {
        (unwired) DB_-_[AMS].[Execute].[Message]_ColNames."[ReceivedOn]" ("[AMS].[Execute].[Message] ColNames")
        (unwired) DB_-_[AMS].[Execute].[Message]_ColNames."[OverallSentStatus]" ("[AMS].[Execute].[Message] ColNames")
        (unwired) DB_-_[AMS].[Execute].[Message]_ColNames."[IsEmailSent]" ("[AMS].[Execute].[Message] ColNames")
        (unwired) DB_-_[AMS].[Execute].[Message]_ColNames."[IsToSendEmail]" ("[AMS].[Execute].[Message] ColNames")
        (unwired) DB_-_[AMS].[Execute].[Message]_ColNames."[IsSmsSent]" ("[AMS].[Execute].[Message] ColNames")
        (unwired) DB_-_[AMS].[Execute].[Message]_ColNames."[IsToSendSms]" ("[AMS].[Execute].[Message] ColNames")
        (unwired) DB_-_[AMS].[Execute].[Message]_ColNames."[MessageLogNo]" ("[AMS].[Execute].[Message] ColNames")
        (unwired) DB_-_[AMS].[Execute].[Message]_ColNames."[MessageNo]" ("[AMS].[Execute].[Message] ColNames")
        (unwired) DB_-_[AMS].[Execute].[Message]_ColNames."[PlantId]" ("[AMS].[Execute].[Message] ColNames")
        (unwired) DB_-_[AMS].[Execute].[Message]_ColNames."[SoftwareSolutionId]" ("[AMS].[Execute].[Message] ColNames")
        # "60s x 60min x 24hrs"
        n167 = event-data() -> ()  [unwired: 1 in, 6 out]
        n168 = property on="Application ComboBox" class="CmbBox (strict)"() -> ("Value"=w332:T2)  [unwired: 2 in, 2 out]
        n169 = property on="Plant" class="CmbBox (strict)"() -> ("Value"=w340:T2)  [unwired: 2 in, 2 out]
        n170 = case shown="\"F\"" "Email" {
          tunnel: ["[IsToSendEmail] = '0'" ("input string") "[IsToSendEmail] = '1' AND [IsEmailSent] = '0'" ("input string") "[IsToSendSms] = '1' AND [IsSmsSent] = '1'" ("input string") "[IsToSendEmail] = '1' AND [IsEmailSent] = '0' AND  [OverallSendStatus] = '0'" ("input string") ""] -> w317
          frame "N" {
          }
          frame "R" {
          }
          frame "S" {
          }
          frame "F" {
          }
          frame "", Default {
          }
        }
        n171 = case shown="\"S\"" "SMS" {
          tunnel: ["[IsToSendSms] = '0'" ("input string") "[IsToSendSms] = '1' AND [IsSmsSent] = '0'" ("input string") "[IsToSendSms] = '1' AND [IsSmsSent] = '1'" ("input string") " [IsToSendSms] = '1' AND [IsSmsSent] = '0' AND  [OverallSendStatus] = '0'" ("input string") ""] -> w319
          frame "N" {
          }
          frame "R" {
          }
          frame "S" {
          }
          frame "F" {
          }
          frame "", Default {
          }
        }
        n172 = Empty String/Path?(string/path=w340) -> (empty?=w343:bool)
        n173 = Empty String/Path?(string/path=w332) -> (empty?=w333:bool)
        n174 = global read "Global AMS.vi" "Date Format"() -> (w313:string)
        n175 = Add(x="To Date", y=86400) -> (x+y=w271:timestamp)
        n176 = Search and Replace String(input string=" [PlantId] = '<PlantId>' AND ", search string="<PlantId>", replace string=w340) -> (result string=w339:string)  [unwired: 5 in, 3 out]
        n177 = Format Date/Time String(time format string (%c)=w313, seconds (now)="From Date") -> (date/time string=w310:string)  [unwired: 1 in]
        n178 = Format Date/Time String(time format string (%c)=w313, seconds (now)=w271) -> (date/time string=w307:string)  [unwired: 1 in]
        n179 = Search and Replace String(input string=" [SoftwareSolutionId] = '<SSID>' AND ", search string="<SSID>", replace string=w332) -> (result string=w336:string)  [unwired: 5 in, 3 out]
        n180 = Select(t="", s=w343, f=w339) -> (s? t:f=w304:string)
        n181 = Select(t="", s=w333, f=w336) -> (s? t:f=w305:string)
        n182 = Search and Replace String(input string=" [ReceivedOn] >= '<FromD>' AND  [ReceivedOn] <= '<ToD>' AND", search string="<FromD>", replace string=w310) -> (result string=w309:string)  [unwired: 5 in, 3 out]
        n183 = Search and Replace String(input string=w309, search string="<ToD>", replace string=w307) -> (result string=w306:string)  [unwired: 5 in, 3 out]
        n184 = Empty String/Path?(string/path=w317) -> (empty?=w321:bool)
        n185 = Empty String/Path?(string/path=w319) -> (empty?=w323:bool)
        n186 = Concatenate Strings(w319, " AND " ("string")) -> (w293:string)
        n187 = Concatenate Strings(w317, " AND " ("string")) -> (w315:string)
        n188 = Select(t="", s=w323, f=w293) -> (s? t:f=w303:string)
        n189 = Select(t="", s=w321, f=w315) -> (s? t:f=w302:string)
        n190 = Number To Decimal String(number="Max Record to Display") -> (decimal integer string=w296:string)  [unwired: 1 in]
        n191 = Search and Replace String(input string=" [MessageNo] LIKE '%<MN>%' AND ", search string="<MN>", replace string="Message No") -> (result string=w301:string)  [unwired: 5 in, 3 out]
        n192 = Search and Replace String(input string=" [MessageLogNo] LIKE '%<ML>%' AND ", search string="<ML>", replace string="Ref Message No") -> (result string=w300:string)  [unwired: 5 in, 3 out]
        n193 = call <vilib>:"Space Constant.vi"() -> ("String"=w295:string)
        n194 = Concatenate Strings("TOP " ("string"), w296, w295) -> (w294:string)
        n195 = Concatenate Strings(w306, w305, w304, w303, w302, w301, w300) -> (w299:string)
        "<CONDITIONS>" <- w299
        n196 = call "DB - [AMS].[Execute].[Message].vi"("<TOP>"=w294, "DB - [AMS].[Execute].[Message] Enum"=DB_-_[AMS].[Execute].[Message]_Enum."SELECT (Multi-Conditions)", "AMS Execute Message ColNames"=w280, "<CONDITIONS>"=w299) -> ("2D data"=w270:string[][], "SUMMARY"=w292:errorcluster)  [unwired: 8 in, 2 out]
        n197 = Search 1D Array(1D array=w280, element=DB_-_[AMS].[Execute].[Message]_ColNames."[SoftwareSolutionId]") -> (index of element=w279:i32)  [unwired: 1 in]
        n198 = Search 1D Array(1D array=w280, element=DB_-_[AMS].[Execute].[Message]_ColNames."[PlantId]") -> (index of element=w285:i32)  [unwired: 1 in]
        n199 = local write "Summary"(w292) -> ()
        n200 = Index Array(array=w270, index (col) #1=w285, index (col) #2=w279) -> (element #1=w284:string[], element #2=w278:string[])  [unwired: 2 in]
        n201 = call "String - Array Group By.vi"("Array in"=w284) -> ("GROUP BY (Array in)"=w282:string[])  [unwired: 10 in]
        n202 = call "String - Array Group By.vi"("Array in"=w278) -> ("GROUP BY (Array in)"=w276:string[])  [unwired: 10 in]
        n203 = Build Array (concatenate)("", w282) -> (w281:string[])
        n204 = Build Array (concatenate)("", w276) -> (w275:string[])
        n205 = property on="Plant" class="CmbBox (strict)"("Strings[]"=w281) -> ()  [unwired: 2 in, 2 out]
        n206 = property on="Application ComboBox" class="CmbBox (strict)"("Strings[]"=w275) -> ()  [unwired: 2 in, 2 out]
        n207 = property on="Multicolumn Listbox" class="MCListbox (strict)"("ItemNames"=w270) -> (error out=w289:errorcluster)  [unwired: 2 in, 1 out]
        n208 = property on="Toggle Refresh MCListBox Colors" class="Bool (strict)"(error in=w289) -> (error out=w288:errorcluster, "Value"=w291:bool)  [unwired: 1 in, 1 out]
        n209 = Not(x=w291) -> (.not. x?=w290:bool)
        n210 = property on="Toggle Refresh MCListBox Colors" class="Bool (strict)"(error in=w288, "Val(Sgnl)"=w290) -> (error out=w287:errorcluster)  [unwired: 1 in, 1 out]
        n211 = local write "Property"(w287) -> ()
      }
      event "Search": Value Change {
        n212 = event-data() -> ()  [unwired: 1 in, 6 out]
        n213 = property on="Toggle Search" class="Bool (strict)"() -> ("Value"=w356:bool)  [unwired: 2 in, 2 out]
        n214 = Not(x=w356) -> (.not. x?=w355:bool)
        n215 = property on="Toggle Search" class="Bool (strict)"("Val(Sgnl)"=w355) -> ()  [unwired: 2 in, 2 out]
      }
      event "Toggle Refresh MCListBox Colors": Value Change {
        w364 = T13 {"Row"=-1, "Column"=-2}  # Col Hdr
        w366 = T13 {"Row"=-2, "Column"=-2}  # Invalid ALL
        # "Reset Color"
        n216 = event-data() -> ()  [unwired: 1 in, 6 out]
        n217 = local read "CellBG Unused Cells"() -> (w365:u32)
        n218 = local read "CellBG ColHdrs"() -> (w363:u32)
        n219 = property on="Multicolumn Listbox" class="MCListbox (strict)"("ActiveCell"=w366, "CellBG"=w365, "ActiveCell"=w364, "CellBG"=w363) -> (error out=w362:errorcluster)  [unwired: 2 in, 1 out]
        n220 = property on="Multicolumn Listbox" class="MCListbox (strict)"(error in=w362) -> (error out=w367:errorcluster, "ItemNames"=w368:string[][])  [unwired: 1 in, 1 out]
        n221 = Search 1D Array(1D array=w360, element=DB_-_[AMS].[Execute].[Message]_ColNames."[IsToSendSms]" ("[AMS].[Execute].[Message] ColNames")) -> (index of element=w377:i32)  [unwired: 1 in]
        n222 = Search 1D Array(1D array=w360, element=DB_-_[AMS].[Execute].[Message]_ColNames."[IsToSendEmail]" ("[AMS].[Execute].[Message] ColNames")) -> (index of element=w372:i32)  [unwired: 1 in]
        n223 = Search 1D Array(1D array=w360, element=DB_-_[AMS].[Execute].[Message]_ColNames."[IsEmailSent]" ("[AMS].[Execute].[Message] ColNames")) -> (index of element=w371:i32)  [unwired: 1 in]
        n224 = Search 1D Array(1D array=w360, element=DB_-_[AMS].[Execute].[Message]_ColNames."[OverallSentStatus]" ("[AMS].[Execute].[Message] ColNames")) -> (index of element=w358:i32)  [unwired: 1 in]
        n225 = Search 1D Array(1D array=w360, element=DB_-_[AMS].[Execute].[Message]_ColNames."[StatusUpdatedOn]" ("[AMS].[Execute].[Message] ColNames")) -> (index of element=w357:i32)  [unwired: 1 in]
        n226 = Search 1D Array(1D array=w360, element=DB_-_[AMS].[Execute].[Message]_ColNames."[IsSmsSent]" ("[AMS].[Execute].[Message] ColNames")) -> (index of element=w375:i32)  [unwired: 1 in]
        n227 = Search 1D Array(1D array=w360, element=DB_-_[AMS].[Execute].[Message]_ColNames."[LastAttemptedOn]" ("[AMS].[Execute].[Message] ColNames")) -> (index of element=w369:i32)  [unwired: 1 in]
        n228 = for {
          tunnel: w368 -> [w386] mode=indexing
          tunnel: w377 -> [w406]
          tunnel: w375 -> [w404]
          tunnel: w372 -> [w402]
          tunnel: w371 -> [w401]
          tunnel: w369 -> [w394]
          tunnel: w367 -> [w388]
          tunnel: w358 -> [w385]
          tunnel: w357 -> [w384]
          i -> [w396]
          n229 = Index Array(array=w386, index #1=w406, index #2=w404, index #3=w402, index #4=w401, index #5=w394) -> (element #1=w405:string, element #2=w403:string, element #3=w400:string, element #4=w399:string, element #5=w389:string)
          n230 = Index Array(array=w386, index #1=w385, index #2=w384) -> (element #1=w381:string, element #2=w383:string)
          n231 = call "DB - Convert BIT Type.vi"("BIT Type (eg Inactive)"=w405) -> ("Boolean"=w393:bool)  [unwired: 2 in, 2 out]
          n232 = call "DB - Convert BIT Type.vi"("BIT Type (eg Inactive)"=w403) -> ("Boolean"=w392:bool)  [unwired: 2 in, 2 out]
          n233 = call "DB - Convert BIT Type.vi"("BIT Type (eg Inactive)"=w400) -> ("Boolean"=w391:bool)  [unwired: 2 in, 2 out]
          n234 = call "DB - Convert BIT Type.vi"("BIT Type (eg Inactive)"=w399) -> ("Boolean"=w390:bool)  [unwired: 2 in, 2 out]
          n235 = call "DB - Convert BIT Type.vi"("BIT Type (eg Inactive)"=w381) -> ("Boolean"=w380:bool)  [unwired: 2 in, 2 out]
          n236 = Empty String/Path?(string/path=w383) -> (empty?=w382:bool)
          n237 = Compound Arithmetic op=AND(w393, w392, w391, w390) -> (w398:bool)
          n238 = case shown="False" w398 {
            tunnel: [w424 u32 6618880] -> _
            tunnel: w393 -> [w423 _]
            tunnel: w392 -> [w422 _]
            tunnel: w391 -> [w420 _]
            tunnel: w390 -> [w419 _]
            tunnel: w389 -> [w415 _]
            frame False {
              # "Blank means not processed"
              n239 = Not(x=w419) -> (.not. x?=w418:bool)
              n240 = Not(x=w422) -> (.not. x?=w421:bool)
              n241 = And(x=w423, y=w421) -> (x .and. y?=w417:bool)
              n242 = And(x=w420, y=w418) -> (x .and. y?=w416:bool)
              n243 = Empty String/Path?(string/path=w415) -> (empty?=w413:bool)
              n244 = Or(x=w417, y=w416) -> (x .or. y?=w414:bool)
              n245 = And(x=w414, y=w413) -> (x .and. y?=w412:bool)
              n246 = case shown="False" w412 {
                tunnel: [u32 16711680 u32 16776770] -> w424
                frame False {
                  # "Processed but still at least one either SMS or EMAIL not sent"
                }
                frame True {
                  # "Requred and not sent"
                }
              }
            }
            frame True {
              # "All SENT"
            }
          }
          n247 = case shown="True" w382 {
            tunnel: [w407 u32 16776770] -> w379
            tunnel: w380 -> [w408 _]
            frame False {
              # "Not empty... Processed"
              n248 = case shown="False" w408 {
                tunnel: [u32 16711680 u32 6618880] -> w407
                frame False {
                }
                frame True {
                }
              }
            }
            frame True {
              # "Empty.. not processed yet"
            }
          }
          n249 = Bundle(w396, 0) -> (w395:cluster{i32, i32})  [unwired: 1 in]
          n250 = property on="Multicolumn Listbox" class="MCListbox (strict)"(error in=w388, "ActiveCell"=w395, "CellBG"=w379, "CellFontColor"=w379) -> (error out=w387:errorcluster)  [unwired: 1 in, 1 out]
          n251 = local write "Property"(w387) -> ()
        }
      }
      event "Excel": Value Change {
        n252 = event-data() -> ()  [unwired: 1 in, 6 out]
        n253 = property on="Multicolumn Listbox" class="MCListbox (strict)"() -> ("ColHdrString"=w435:string[], "ItemNames"=w434:string[][])  [unwired: 2 in, 2 out]
        n254 = call "File Dialog"("prompt"="Excel File Path") -> ("selected path"=w431:path, "error out"=w429:errorcluster)  [unwired: 11 in, 2 out]
        n255 = call <vilib>:"New Report.vi"("window state (normal)"=T21."minimized", "report type"=T22."Excel", "error in (no error)"=w429) -> ("report out"=w444:refnum<class "NI_report.lvclass">, "error out"=w443:errorcluster)  [unwired: 11 in]
        n256 = call-poly <vilib>:"Append Table to Report.vi"("report in"=w444, "column headers"=w435, "text data"=w434, "error in (no error)"=w443) -> ("report out"=w442:refnum<class "NI_report.lvclass">, "error out"=w441:errorcluster)  [unwired: 8 in, 2 out]
        n257 = call-dynamic "Save Report to File.vi"("report in"=w442, "report file path"=w431, "prompt to replace? (F)"=TRUE, "error in (no error)"=w441) -> ("report out"=w440:refnum<class "NI_report.lvclass">, "error out"=w439:errorcluster)  [unwired: 10 in]
        n258 = call-dynamic "Dispose Report.vi"("report in"=w440, "wait until printing completed? (T)"=FALSE, "save changes? (F)"=FALSE, "error in (no error)"=w439) -> ("error out"=→"Report":errorcluster)  [unwired: 11 in]
      }
      event "Resend": Value Change {
        n259 = event-data() -> ()  [unwired: 1 in, 6 out]
        n260 = property on="Multicolumn Listbox" class="MCListbox (strict)"() -> ("Value"=w445:i32[])  [unwired: 2 in, 2 out]
        n261 = Array Size(array=w445) -> (size(s)=w446:i32)
        n262 = Search 1D Array(1D array=w450, element=DB_-_[AMS].[Execute].[Message]_ColNames."[MessageNo]") -> (index of element=w448:i32)  [unwired: 1 in]
        n263 = Greater Or Equal To 0?(x=w446) -> (x >= 0?=w447:bool)
        n264 = case shown="True" w447 {
          tunnel: w448 -> [_ w456]
          tunnel: w445 -> [_ w455]
          frame False {
          }
          frame True {
            n265 = for {
              tunnel: w456 -> [w461]
              tunnel: w455 -> [w460] mode=indexing
              shift-right: [w457] -> w453
              shift-left: errorcluster {"status"=FALSE, "code"=0, "source"=""} ("SUMMARY") -> [w458]
              # "RE-INSERT one by one"
              n266 = property on="Multicolumn Listbox" class="MCListbox (strict)"() -> ("ItemNames"=w462:string[][])  [unwired: 2 in, 2 out]
              n267 = Index Array(array=w462, index (row)=w460, index (col)=w461) -> (element=w459:string)
              n268 = call "DB - [AMS].[Execute].[Message].vi"("DB - [AMS].[Execute].[Message] Enum"=DB_-_[AMS].[Execute].[Message]_Enum."RE-INSERT", "error in (no error)"=w458, "[MessageNo]"=w459) -> ("SUMMARY"=w457:errorcluster)  [unwired: 9 in, 3 out]
            }
            "Summary" <- w453
            n269 = property on="Multicolumn Listbox" class="MCListbox (strict)"(error in=w453, "Value"=i32[] [] ("Multicolumn Listbox")) -> (error out=→"Property":errorcluster)  [unwired: 1 in, 1 out]
          }
        }
      }
    }
    "Close Flag" <- w90
  }
  n270 = while {
    tunnel: w5 -> [w471]
    shift-right: [w467] -> _
    shift-left: w4 -> [w470]
    tunnel: [w464] -> w3
    stop <- w464 stop-if-true
    w468 = Enum_-_CMS_State."QUIT"  # CMS Main Process
    # "StateMachine For MainProcess                                                                                             StateMachine For MainProcess                                                                                             StateMachine For MainProcess                                                                                             StateMachine For MainProcess                                                                                             StateMachine For MainProcess                                                                                             StateMachine For MainProcess                                                                                             StateMachine For MainProcess"
    n271 = case shown="\"READY TO START\", Default" w470 {
      selector: w470 -> [w472 w567 w598]
      tunnel: w471 -> [_ w568 _]
      tunnel: [_ _ TRUE] -> w464
      tunnel: [w473 w566 w598] -> w466
      frame "READY TO START", Default {
        n272 = local read "Tab Body"() -> (w474:T1)
        n273 = case shown="\"Logon\"" w474 {
          tunnel: [w475 w477] -> w473
          tunnel: w472 -> [w475 w476]
          frame Default {
          }
          frame "Logon" {
            n274 = local read "Logon OK"() -> (w478:bool)
            n275 = case shown="True" w478 {
              tunnel: [w479 w546] -> w477
              tunnel: w476 -> [w479 _]
              frame False {
                # "Not Logon Yet"
                n276 = flat-sequence {
                  tunnel: [w484] -> w480
                  tunnel: [w493] -> w482
                  tunnel: [w492] -> w481
                  tunnel: w480 -> [w492]
                  tunnel: w482 -> [w495]
                  tunnel: w481 -> [w494]
                  frame #0 {
                    n277 = local read "Logon UI"() -> (w484:refnum<vi>)
                    n278 = control-ref of="Logon OK"() -> (w483:refnum<vi>)
                    n279 = control-ref of="Logon"() -> (w487:refnum<vi>)
                    n280 = control-ref of="Logon Extra"() -> (w486:refnum<vi>)
                    n281 = control-ref of="[TabUserAccess]"() -> (w485:refnum<vi>)
                    n282 = Build Array(w483, w487, w486, w485) -> (w488:refnum<vi>[])
                    n283 = for {
                      tunnel: w484 -> [w491]
                      tunnel: w488 -> [w490] mode=indexing
                      n284 = call "subPanel - Read Value.vi"("subPanel Ref"=w491, "CtlRef"=w490) -> ("Error Out"=w489:errorcluster)  [unwired: 6 in, 3 out]
                      n285 = local write "SubPanel Error"(w489) -> ()
                    }
                  }
                  frame #1 {
                    n286 = local read "Logon OK"() -> (w493:bool)
                  }
                  frame #2 {
                    n287 = case shown="True" w495 {
                      tunnel: w494 -> [_ w499]
                      frame False {
                      }
                      frame True {
                        # "Logon UI should already be closed"
                        n288 = control-ref of="Logon UI"() -> (w498:refnum<vi>)
                        n289 = Close Reference(reference=w499) -> (error out=w500:errorcluster)  [unwired: 1 in]
                        n290 = invoke on="Invoke Node" class="SubPnl" method="Remove VI"(reference=w498, error in=w500) -> ()  [unwired: 1 in, 3 out]
                        n291 = global write "Global AMS.vi" "Logon Extra"("Logon Extra") -> ()
                        n292 = global write "Global AMS.vi" "Logon"("Logon") -> ()
                      }
                    }
                  }
                }
              }
              frame True {
                w510 = TRUE ("write raw string? (F)")
                w509 = "Settings" ("section")
                w537 = 5  # [CmsServerTz]
                w545 = 1  # [TimeZone]
                w544 = 2  # [Software Solution Description]
                w543 = 0  # [LogoFile]
                w546 = Enum_-_CMS_State."RUNNING Process"  # StateMachine for CMS Main Process
                # "Logon OK"
                n293 = flat-sequence {
                  tunnel: [w548] -> w526
                  frame #0 {
                    # "Last to Show. Otherwise will Fliker through all Tabs"
                    n294 = local read "Show Debug TAB"() -> (w549:bool)
                    n295 = property on="Tab Body" class="TabCtl (strict)"() -> ("Pages"=w550:refnum<vi>[])  [unwired: 2 in, 2 out]
                    n296 = for {
                      tunnel: w550 -> [w556] mode=indexing
                      tunnel: w549 -> [w555]
                      tunnel: [w551] -> w548
                      n297 = property class="Page"(reference=w556) -> (reference out=w552:refnum<vi>, "PageLabel"=w554:string)  [unwired: 1 in, 1 out]
                      n298 = case shown="\"Debug\"" w554 {
                        tunnel: w555 -> [_ w558 _ _]
                        tunnel: [FALSE ("Show Debug TAB") w558 FALSE TRUE] -> w553
                        frame Default {
                        }
                        frame "Debug" {
                          # "Debug dependent of \n\"Show Report Tab ONLY\""
                        }
                        frame "Logon" {
                        }
                        frame "WIN1", "WIN8" {
                          # "These Tabs ALWAYS shown"
                        }
                      }
                      n299 = property class="Page"(reference=w552, "PageVis"=w553) -> (reference out=w551:refnum<vi>)  [unwired: 1 in, 1 out]
                    }
                  }
                }
                n300 = global read "Global AMS.vi" "Logon"() -> (w522:T5)
                n301 = global read "Global CMS.vi" "Logon Extra"() -> (w531:T4)
                n302 = Unbundle By Name(w522) -> ("PlantID"=w538:string, "LanguageID"=w525:string)
                n303 = call "DB - [Config].[SoftwareSolution].vi"("[LanguageId]"=w525, "Application"="AMS", "[PlantId]"=w538) -> ("1D data"=w542:string[])  [unwired: 6 in, 2 out]
                n304 = Unbundle By Name(w531) -> ("Plant Name"=w530:string, "UserName"=w528:string)
                n305 = Index Array(array=w542, index #1=w543, index #2=w545, index #3=w544, index #4=w537) -> (element #1=w505:string, element #2=w536:string, element #3=w504:string, element #4=w535:string)
                "[TimeZone] (Plant)" <- w536
                "[CmsServerTz] (CMS)" <- w535
                n306 = String To Path(string=w505) -> (path=w541:path)
                n307 = call <vilib>:"Read JPEG File.vi"("path to JPEG file"=w541) -> ("error out"=w521:errorcluster, "image data"=w540:T17)  [unwired: 8 in, 1 out]
                n308 = Concatenate Strings(w530, ", " ("string"), w528) -> (w527:string)
                n309 = property on="Close" class="Bool (strict)"("BoolText.Text"="Log off") -> ()  [unwired: 2 in, 2 out]
                n310 = call <vilib>:"Draw Flattened Pixmap.vi"("image data"=w540) -> ("new picture"=w520:picture)  [unwired: 8 in]
                n311 = control-ref of="ApplicationName"() -> (w524:refnum<vi>)
                n312 = local write "Plant and Furnace Name"(w527) -> ()
                n313 = call <vilib>:"Application Directory.vi"() -> ("Application Directory"=w518:path)
                n314 = call "Tool_Unicode Update String.vi"("Interpret as Unicode (T)"=TRUE, "String Value"=w504, "String Control Reference"=w524) -> ()  [unwired: 5 in, 2 out]
                n315 = Build Path(base path=w518, name or relative path="AMSClient.ini" ("ini Name")) -> (appended path=w515:path)
                n316 = local write "LogonName Error"(w521) -> ()
                n317 = local write "LogoName"(w520) -> ()
                n318 = Decimal String To Number(string=w536) -> (number=w533:i32)  [unwired: 2 in, 1 out]
                n319 = Decimal String To Number(string=w535) -> (number=w534:i32)  [unwired: 2 in, 1 out]
                n320 = call <vilib>:"Open Config Data.vi"("create file if necessary (T)"=FALSE, "configuration file path"=w515) -> ("error out"=w513:errorcluster, "refnum"=w514:T26)  [unwired: 7 in, 1 out]
                n321 = Subtract(x=w534, y=w533) -> (x-y=w502:i32)
                "TimeZone Diff (NA)" <- w502
                n322 = flat-sequence {
                  tunnel: w526 -> [_]
                  tunnel: [T1."Monitor" ("Tab Body")] -> w501
                  frame #0 {
                    # "Only settable Tabs\nare listed\nDebug, Logon\nControlled by App\nso not listed here"
                    n323 = control-ref of="Tab Body"() -> (w564:refnum<vi>)
                    n324 = call "Tabs - Page Visibility.vi"("Matching Tab#"=i32[] [0, 11, 12], "PageLabel"=string[] ["Monitor", "Admin", "Config"], "[TabUserAccess]"="[TabUserAccess]", "TabControl in"=w564) -> ()  [unwired: 7 in, 1 out]
                  }
                }
                n325 = call-poly <vilib>:"Write Key.vi"("write raw string? (F)"=w510, "section"=w509, "error in (no error)"=w513, "value"=w505, "key"="LogoFile", "refnum"=w514) -> ("error out"=w511:errorcluster, "refnum out"=w512:T26)  [unwired: 3 in, 1 out]
                n326 = call-poly <vilib>:"Write Key.vi"("write raw string? (F)"=w510, "section"=w509, "error in (no error)"=w511, "value"=w504, "key"="Software Solution Name", "refnum"=w512) -> ("error out"=w507:errorcluster, "refnum out"=w506:T26)  [unwired: 3 in, 1 out]
                n327 = call <vilib>:"Close Config Data.vi"("error in (no error)"=w507, "refnum"=w506) -> ("error out"=w503:errorcluster)  [unwired: 8 in, 1 out]
                n328 = local write "ini File"(w503) -> ()
                n329 = flat-sequence {
                  tunnel: w503 -> [_]
                  tunnel: w502 -> [_]
                  tunnel: w501 -> [_]
                  frame #0 {
                    n330 = property on="Toggle Search" class="Bool (strict)"("Val(Sgnl)"=TRUE) -> ()  [unwired: 2 in, 2 out]
                  }
                }
                n331 = property on="Tab Body" class="TabCtl (strict)"("Val(Sgnl)"=w501) -> ()  [unwired: 2 in, 2 out]
              }
            }
          }
        }
      }
      frame "RUNNING Process" {
        n332 = while {
          tunnel: w568 -> [_]
          tunnel: w567 -> [w575]
          tunnel: [w574] -> w566
          stop <- w577 stop-if-true
          w573 = Enum_-_CMS_State."READY TO START"  # CMS Main Process
          n333 = Format Date/Time String(time format string (%c)="%b %d, %Y  %H:%M:%S") -> (date/time string=→"Current Time":string)  [unwired: 2 in]
          n334 = call "Elapsed Time"("Time Target (s)"="Time Target (s)") -> ("Time has Elapsed"=w571:bool)  [unwired: 11 in, 7 out]
          n335 = Wait Until Next ms Multiple(millisecond multiple=u32 100) -> ()  [unwired: 1 out]
          n336 = case shown="True" w571 {
            frame False {
            }
            frame True {
              w591 = DB_-_[AMS].[Execute].[EventLog]_Enum."SELECT 'CreatedOn'" ("DB - [AMS].[Execute].[EventLog]")
              n337 = local read "EnginePollIntInSec"() -> (w597:i32)
              n338 = call "DB - [AMS].[Execute].[EventLog].vi"("DB - [AMS].[Execute].[EventLog]"=w591, "DB Connection"=T25 {"Open"=TRUE, "Close"=FALSE}, "AMS Execute EventLog"=T24 {"EventType"="Start", "Source"="Engine", "UserId"="AMSServer", "Computer"="", "CreatedOn"="", "Remarks1"=""}) -> ("time stamp"=w582:timestamp, "connection reference"=w596:T28)  [unwired: 4 in, 3 out]
              "Engine Start" <- w582
              n339 = local write "Time Target (s)"(w597) -> ()
              n340 = call "DB - [AMS].[Execute].[EventLog].vi"("DB - [AMS].[Execute].[EventLog]"=w591, "DB Connection"=T25 {"Open"=FALSE, "Close"=FALSE}, "AMS Execute EventLog"=T24 {"EventType"="Alive", "Source"="Engine", "UserId"="AMSServer", "Computer"="", "CreatedOn"="", "Remarks1"=""}, "connection reference"=w596) -> ("time stamp"=w587:timestamp, "[CreatedOn]"=w583:string, "connection reference"=w595:T28)  [unwired: 3 in, 2 out]
              "Engine Alive" <- w587
              n341 = call "DB - [AMS].[Execute].[EventLog].vi"("DB - [AMS].[Execute].[EventLog]"=w591, "DB Connection"=T25 {"Open"=FALSE, "Close"=TRUE}, "AMS Execute EventLog"=T24 {"EventType"="Stop", "Source"="Engine", "UserId"="AMSServer", "Computer"="", "CreatedOn"="", "Remarks1"=""}, "connection reference"=w595) -> ("time stamp"=w581:timestamp)  [unwired: 3 in, 4 out]
              "Engine Stop" <- w581
              n342 = Greater?(x=w587, y=w582) -> (0:w586:bool)
              n343 = Greater?(x=w587, y=w581) -> (0:w585:bool)
              n344 = And(x=w586, y=w585) -> (x .and. y?=w584:bool)
              n345 = local write "Overall Status"(w584) -> ()
              n346 = local write "Last Alive On"(w583) -> ()
            }
          }
          n347 = local read "Logon OK"() -> (w576:bool)
          n348 = local read "Close Flag"() -> (w579:bool)
          n349 = Not(x=w576) -> (.not. x?=w578:bool)
          n350 = Or(x=w578, y=w579) -> (x .or. y?=w577:bool)
          n351 = Select "Check if User Log off"(t=w575, s=w576, f=w573) -> (s? t:f=w574:T8)
        }
      }
      frame "QUIT" {
      }
    }
    n352 = Wait Until Next ms Multiple(millisecond multiple=u32 100) -> ()  [unwired: 1 out]
    n353 = local read "Quit Flag"() -> (w469:bool)
    n354 = Select(t=w468, s=w469, f=w466) -> (s? t:f=w467:T8)
  }
  n355 = flat-sequence {
    tunnel: w3 -> [_]
    tunnel: w2 -> [_]
    frame #0 {
      n356 = local read "Application:Name"() -> (w605:string)
      n357 = To Upper Case(1:w605) -> (0:w604:string)
      n358 = To Upper Case(1:"LabVIEW.exe" ("regular expression")) -> (0:w602:string)
      n359 = Match Pattern(string=w604, regular expression=w602) -> (offset past match=w601:i32)  [unwired: 1 in, 3 out]
      n360 = Greater Or Equal To 0?(x=w601) -> (x >= 0?=w600:bool)
      n361 = case shown="True" w600 {
        frame False {
          # "Executable"
          n362 = control-ref of="This VI"() -> (w606:refnum<vi>)
          n363 = invoke class="VI" method="FP.Close"(reference=w606) -> ()  [unwired: 2 in, 3 out]
        }
        frame True {
          # "Show Debug TAB"
          # "LabVIEW Development"
          n364 = property on="Tab Body" class="TabCtl (strict)"() -> ("Pages"=w607:refnum<vi>[])  [unwired: 2 in, 2 out]
          n365 = for {
            tunnel: w607 -> [w612] mode=indexing
            n366 = property class="Page"(reference=w612) -> (reference out=w608:refnum<vi>, "PageLabel"=w611:string)  [unwired: 1 in, 1 out]
            n367 = Equal?(x=w611, y="Debug") -> (x = y?=w609:bool)
            n368 = case shown="True" w609 {
              tunnel: w608 -> [_ w614]
              frame False {
              }
              frame True {
                n369 = property class="Page"(reference=w614, "PageVis"=TRUE) -> ()  [unwired: 1 in, 2 out]
              }
            }
          }
        }
      }
    }
  }
